vi "数据编码.vi"(0 "table输入":string(combo), 1 "仪器参数上传时间":enum16{"精确到小时", "原始时间"}(ring), 5 "错误常量 2":errorcluster caption="错误输入", 7 "仪器参数":string[](array[string]), 9 "QN":string, 11 "参数":string, 13 "MN":string, 14 "PW":string) -> (4 "错误常量":errorcluster caption="错误输出", 15 "通讯包字符串":string)   [LabVIEW 2016, in "数据传输系统-05.lvlib"]
panel:
  out "核查数据发送次数":i32
  out "小时数据发送次数":i32
  out "长度":i32
  in  "数据块":T1
  out "通讯包":T2={"包头（2）"="##", "数据段长度（4）"="", "数据段"="", "CRC校验"="", "包尾"=""}
  # "范例代码：\n\n##0101QN=20160801085857223;ST=32;CN=1062;PW=100000;MN=010000A8900016F000169DC0;Flag=5\n;CP=&&RtdInterval=30&&1C80\\r\\n"
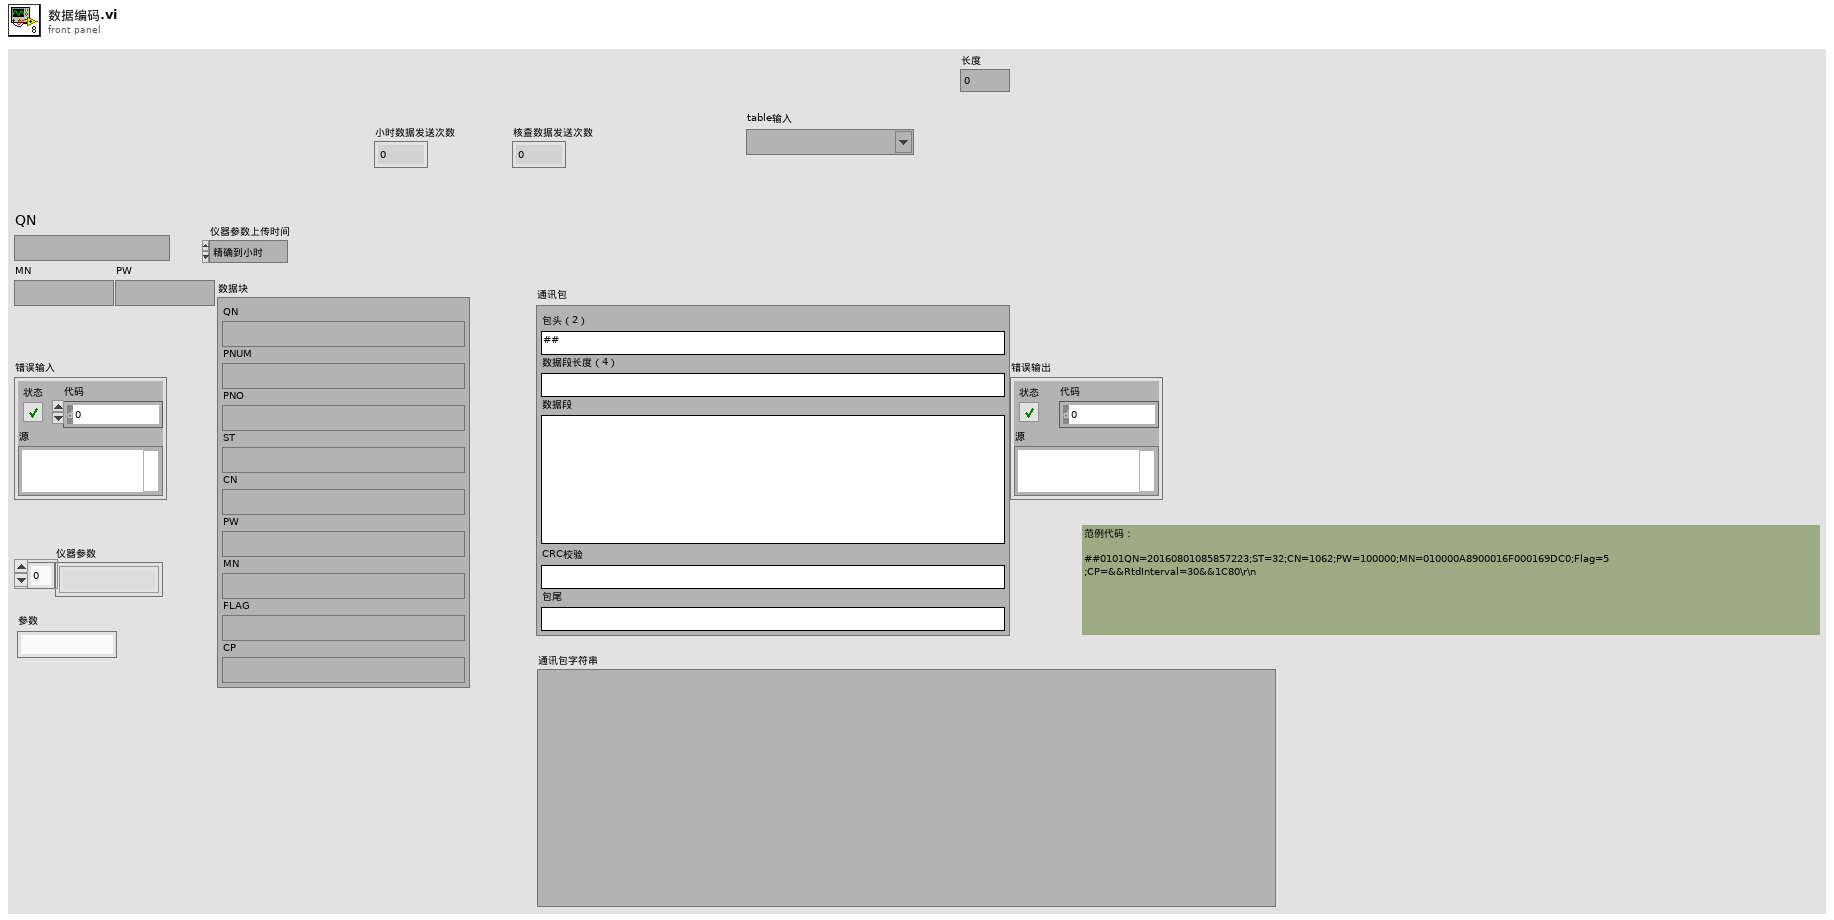
[diagram p1: front panel]
types:
  T1 = cluster{"QN":string, "ST":string, "CN":string, "PW":string, "MN":string, "FLAG":string, "PNUM":string, "PNO":string, "CP":string}
  T2 = cluster{"包头（2）":string, "数据段长度（4）":string, "数据段":string, "CRC校验":string, "包尾":string}
  T3 = cluster{"PH":string[][], "CODCr":string[][], "氨氮":string[][], "CODMn":string[][], "总氮":string[][], "总磷":string[][], "电导率":string[][], "水温":string[][], "DO":string[][], "浊度":string[][], "叶绿素":string[][], "藻密度":string[][], "铜":string[][], "盐度":string[][], "水位":string[][], "流速":string[][], "瞬时流量":string[][], "累积流量":string[][], "亚硝酸盐":string[][], "硫化物":string[][], "ORP":string[][], "铅":string[][], "镉":string[][], "锌":string[][], "镍":string[][], "锰":string[][], "汞":string[][], "气温":string[][], "气压":string[][], "风速":string[][], "风向":string[][], "盐度 2":string[][], "磷酸盐":string[][], "硝氮":string[][], "氟化物":string[][]}
  T4 = enum16{"小时数据", "实时数据", "平行样测试", "集成干预测试", "加标回收测试", "核查数据", "空白零点跨度数据", "提取小时数据", "提取实时数据"}
  T5 = enum16{"小时数据", "实时数据", "平行样测试", "集成干预测试", "加标回收测试", "核查数据", "空白零点跨度数据", "提取小时数据", "提取实时数据", "操作日志"}
  T6 = enum16{"小时数据", "实时数据", "平行样测试", "集成干预测试", "加标回收测试", "核查数据", "空白零点跨度数据", "提取小时数据", "提取实时数据", "操作日志", "仪器参数", "3090仪器参数", "提取仪器参数", "报警信息"}
  T7 = cluster{"CODMn":string, "CODCr":string, "DO":string, "铜":string, "PH":string, "氨氮":string, "比电导率":string, "水温":string, "COD":string, "浊度":string, "总氮":string, "总磷":string, "叶绿素a":string, "藻密度":string, "水位":string, "流速":string, "瞬时流量":string, "累积流量":string, "亚硝酸盐":string, "硫化物":string, "ORP":string, "铅":string, "镉":string, "锌":string, "镍":string, "锰":string, "汞":string, "气温":string, "气压":string, "风速":string, "风向":string, "盐度":string, "磷酸盐":string, "硝氮":string, "氟化物":string}
  T8 = cluster{"CODMn":dbl, "CODCr":dbl, "DO":dbl, "铜":dbl, "PH":dbl, "氨氮":dbl, "比电导率":dbl, "水温":dbl, "COD":dbl, "浊度":dbl, "总氮":dbl, "总磷":dbl, "叶绿素a":dbl, "藻密度":dbl, "水位":dbl, "流速":dbl, "瞬时流量":dbl, "累积流量":dbl, "亚硝酸盐":dbl, "硫化物":dbl, "ORP":dbl, "铅":dbl, "镉":dbl, "锌":dbl, "镍":dbl, "锰":dbl, "汞":dbl, "气温":dbl, "气压":dbl, "风速":dbl, "风向":dbl, "盐度":dbl, "磷酸盐":dbl, "硝氮":dbl, "氟化物":dbl}
  T9 = typedef "LVDateTimeRec.ctl" = cluster{"秒数的小数部分":dbl, "秒":i32, "分":i32, "时":i32, "日":i32, "月":i32, "年":i32, "天数（周）":i32, "天数（年）":i32, "DST":i32}
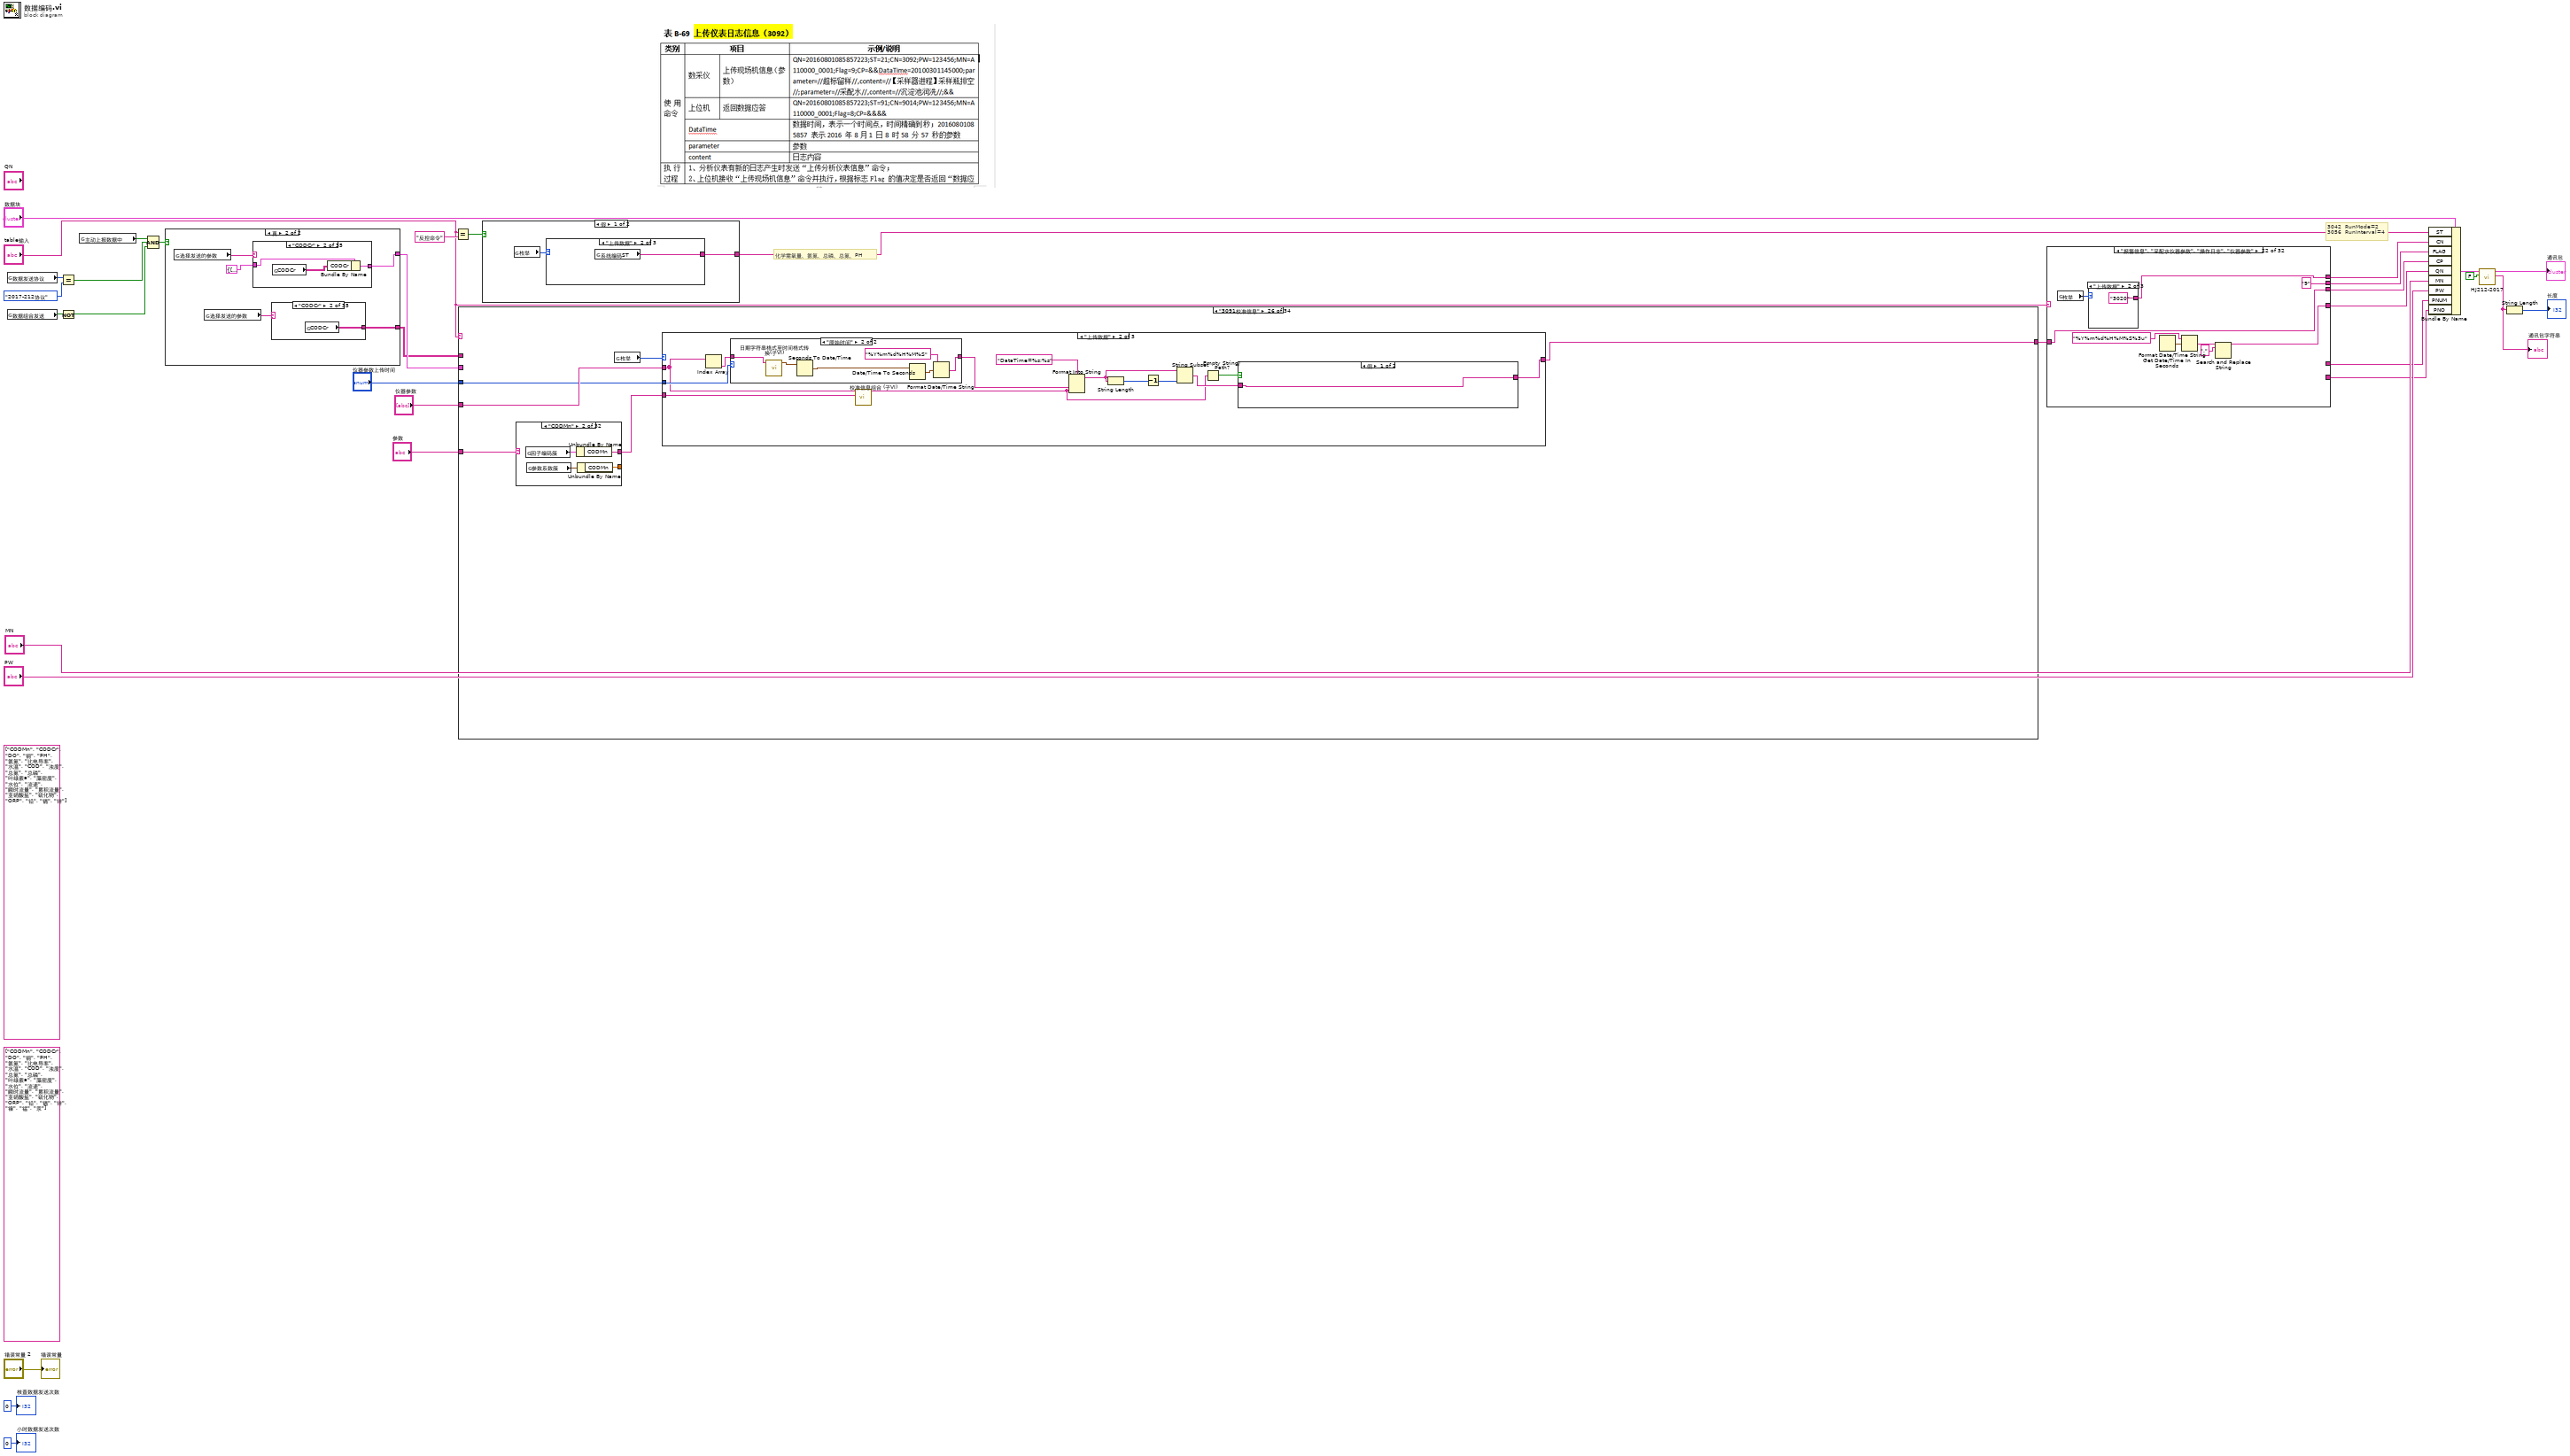
[diagram p0: block diagram]
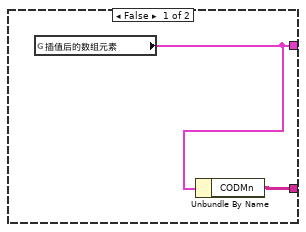
[diagram p2: hidden frame]
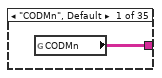
[diagram p3: hidden frame]
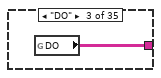
[diagram p4: hidden frame]
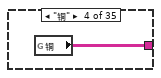
[diagram p5: hidden frame]
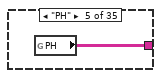
[diagram p6: hidden frame]
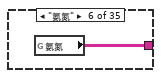
[diagram p7: hidden frame]
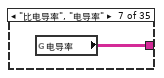
[diagram p8: hidden frame]
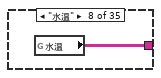
[diagram p9: hidden frame]
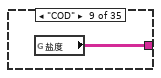
[diagram p10: hidden frame]
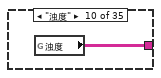
[diagram p11: hidden frame]
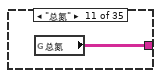
[diagram p12: hidden frame]
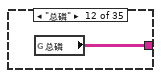
[diagram p13: hidden frame]
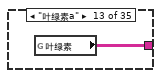
[diagram p14: hidden frame]
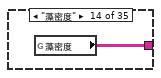
[diagram p15: hidden frame]
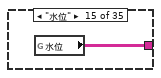
[diagram p16: hidden frame]
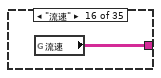
[diagram p17: hidden frame]
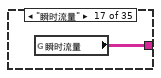
[diagram p18: hidden frame]
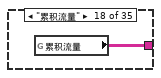
[diagram p19: hidden frame]
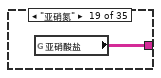
[diagram p20: hidden frame]
diagram:
  (unwired) string[] ["CODMn", "CODCr", "DO", "铜", "PH", "氨氮", "比电导率", "水温", "COD", "浊度", "总氮", "总磷", "叶绿素a", "藻密度", "水位", "流速", "瞬时流量", "累积流量", "亚硝酸盐", "硫化物", "ORP", "铅", "镉", "锌"] ("数组")
  (unwired) string[] ["CODMn", "CODCr", "DO", "铜", "PH", "氨氮", "比电导率", "水温", "COD", "浊度", "总氮", "总磷", "叶绿素a", "藻密度", "水位", "流速", "瞬时流量", "累积流量", "亚硝酸盐", "硫化物", "ORP", "铅", "镉", "锌", "镍", "锰", "汞"] ("数组")
  # "化学需氧量、氨氮、总磷、总氮、PH"
  # "3042  RunMode=2\n3056  RunInterval=4"
  n1 = global read "断电保存全局.vi" "数据发送协议"() -> (w11:enum16{"2005-212协议", "2017-212协议"})
  n2 = global read "断电保存全局.vi" "数据组合发送"() -> (w13:bool)
  n3 = Equal?(x=w11, y=enum16{"2005-212协议", "2017-212协议"}."2017-212协议" ("数据发送版本")) -> (x = y?=w14:bool)
  n4 = Not(x=w13) -> (.not. x?=w12:bool)
  n5 = global read "全局 数据发送重叠.vi" "主动上报数据中"() -> (w18:bool)
  n6 = Compound Arithmetic op=AND ("复合运算")(w18, w14, w12) -> (w15:bool)
  n7 = case shown="真" w15 {
    tunnel: [w36 w40] -> w9
    tunnel: [w35 w38] -> w7
    frame False {
      n8 = global read "插值后的新数组.vi" "插值后的数组元素"() -> (w36:T3)
      n9 = Unbundle By Name(w36) -> ("CODMn"=w35:string[][])
    }
    frame True {
      n10 = global read "全局 水样时间.vi" "选择发送的参数"() -> (w41:string)
      n11 = global read "全局 水样时间.vi" "选择发送的参数"() -> (w39:string)
      n12 = case shown="\"CODCr\"" w41 {
        tunnel: T3 {"PH"=[], "CODCr"=[], "氨氮"=[], "CODMn"=[], "总氮"=[], "总磷"=[], "电导率"=[], "水温"=[], "DO"=[], "浊度"=[], "叶绿素"=[], "藻密度"=[], "铜"=[], "盐度"=[], "水位"=[], "流速"=[], "瞬时流量"=[], "累积流量"=[], "亚硝酸盐"=[], "硫化物"=[], "ORP"=[], "铅"=[], "镉"=[], "锌"=[], "镍"=[], "锰"=[], "汞"=[], "气温"=[], "气压"=[], "风速"=[], "风向"=[], "盐度 2"=[], "磷酸盐"=[], "硝氮"=[], "氟化物"=[]} ("插值后的数组元素") -> [w78 w82 w85 w88 w91 w94 w97 w100 w103 w106 w109 w112 w115 w117 w121 w124 w126 w129 w132 w135 w138 w141 w144 w147 w150 w153 w156 w159 w162 w165 w168 w171 w174 w177 w180]
        tunnel: [w77 w80 w83 w86 w89 w92 w96 w99 w101 w104 w107 w110 w113 w116 w119 w122 w125 w128 w131 w134 w137 w140 w143 w146 w149 w152 w155 w158 w161 w164 w167 w170 w173 w176 w179] -> w40
        frame "CODMn", Default {
          n13 = global read "全局 所有参数.vi" "CODMn"() -> (w79:string[][])
          n14 = Bundle By Name(cluster=w78, "CODMn"=w79) -> (w77:T3)
        }
        frame "CODCr" {
          n15 = global read "全局 所有参数.vi" "CODCr"() -> (w81:string[][])
          n16 = Bundle By Name(cluster=w82, "CODCr"=w81) -> (w80:T3)
        }
        frame "DO" {
          n17 = global read "全局 所有参数.vi" "DO"() -> (w84:string[][])
          n18 = Bundle By Name(cluster=w85, "DO"=w84) -> (w83:T3)
        }
        frame "铜" {
          n19 = global read "全局 所有参数.vi" "铜"() -> (w87:string[][])
          n20 = Bundle By Name(cluster=w88, "铜"=w87) -> (w86:T3)
        }
        frame "PH" {
          n21 = global read "全局 所有参数.vi" "PH"() -> (w90:string[][])
          n22 = Bundle By Name(cluster=w91, "PH"=w90) -> (w89:T3)
        }
        frame "氨氮" {
          n23 = global read "全局 所有参数.vi" "氨氮"() -> (w93:string[][])
          n24 = Bundle By Name(cluster=w94, "氨氮"=w93) -> (w92:T3)
        }
        frame "比电导率", "电导率" {
          n25 = global read "全局 所有参数.vi" "电导率"() -> (w95:string[][])
          n26 = Bundle By Name(cluster=w97, "电导率"=w95) -> (w96:T3)
        }
        frame "水温" {
          n27 = global read "全局 所有参数.vi" "水温"() -> (w98:string[][])
          n28 = Bundle By Name(cluster=w100, "水温"=w98) -> (w99:T3)
        }
        frame "COD" {
          n29 = global read "全局 所有参数.vi" "盐度"() -> (w102:string[][])
          n30 = Bundle By Name(cluster=w103, "盐度"=w102) -> (w101:T3)
        }
        frame "浊度" {
          n31 = global read "全局 所有参数.vi" "浊度"() -> (w105:string[][])
          n32 = Bundle By Name(cluster=w106, "浊度"=w105) -> (w104:T3)
        }
        frame "总氮" {
          n33 = global read "全局 所有参数.vi" "总氮"() -> (w108:string[][])
          n34 = Bundle By Name(cluster=w109, "总氮"=w108) -> (w107:T3)
        }
        frame "总磷" {
          n35 = global read "全局 所有参数.vi" "总磷"() -> (w111:string[][])
          n36 = Bundle By Name(cluster=w112, "总磷"=w111) -> (w110:T3)
        }
        frame "叶绿素a" {
          n37 = global read "全局 所有参数.vi" "叶绿素"() -> (w114:string[][])
          n38 = Bundle By Name(cluster=w115, "叶绿素"=w114) -> (w113:T3)
        }
        frame "藻密度" {
          n39 = global read "全局 所有参数.vi" "藻密度"() -> (w118:string[][])
          n40 = Bundle By Name(cluster=w117, "藻密度"=w118) -> (w116:T3)
        }
        frame "水位" {
          n41 = global read "全局 所有参数.vi" "水位"() -> (w120:string[][])
          n42 = Bundle By Name(cluster=w121, "水位"=w120) -> (w119:T3)
        }
        frame "流速" {
          n43 = global read "全局 所有参数.vi" "流速"() -> (w123:string[][])
          n44 = Bundle By Name(cluster=w124, "流速"=w123) -> (w122:T3)
        }
        frame "瞬时流量" {
          n45 = global read "全局 所有参数.vi" "瞬时流量"() -> (w127:string[][])
          n46 = Bundle By Name(cluster=w126, "瞬时流量"=w127) -> (w125:T3)
        }
        frame "累积流量" {
          n47 = global read "全局 所有参数.vi" "累积流量"() -> (w130:string[][])
          n48 = Bundle By Name(cluster=w129, "累积流量"=w130) -> (w128:T3)
        }
        frame "亚硝氮" {
          n49 = global read "全局 所有参数.vi" "亚硝酸盐"() -> (w133:string[][])
          n50 = Bundle By Name(cluster=w132, "亚硝酸盐"=w133) -> (w131:T3)
        }
        frame "硫化物" {
          n51 = global read "全局 所有参数.vi" "硫化物"() -> (w136:string[][])
          n52 = Bundle By Name(cluster=w135, "硫化物"=w136) -> (w134:T3)
        }
        frame "ORP" {
          n53 = global read "全局 所有参数.vi" "ORP"() -> (w139:string[][])
          n54 = Bundle By Name(cluster=w138, "ORP"=w139) -> (w137:T3)
        }
        frame "铅" {
          n55 = global read "全局 所有参数.vi" "铅"() -> (w142:string[][])
          n56 = Bundle By Name(cluster=w141, "铅"=w142) -> (w140:T3)
        }
        frame "镉" {
          n57 = global read "全局 所有参数.vi" "镉"() -> (w145:string[][])
          n58 = Bundle By Name(cluster=w144, "镉"=w145) -> (w143:T3)
        }
        frame "锌" {
          n59 = global read "全局 所有参数.vi" "锌"() -> (w148:string[][])
          n60 = Bundle By Name(cluster=w147, "锌"=w148) -> (w146:T3)
        }
        frame "镍" {
          n61 = global read "全局 所有参数.vi" "镍"() -> (w151:string[][])
          n62 = Bundle By Name(cluster=w150, "镍"=w151) -> (w149:T3)
        }
        frame "锰" {
          n63 = global read "全局 所有参数.vi" "锰"() -> (w154:string[][])
          n64 = Bundle By Name(cluster=w153, "锰"=w154) -> (w152:T3)
        }
        frame "汞" {
          n65 = global read "全局 所有参数.vi" "汞"() -> (w157:string[][])
          n66 = Bundle By Name(cluster=w156, "汞"=w157) -> (w155:T3)
        }
        frame "气温" {
          n67 = global read "全局 所有参数.vi" "气温"() -> (w160:string[][])
          n68 = Bundle By Name(cluster=w159, "气温"=w160) -> (w158:T3)
        }
        frame "气压" {
          n69 = global read "全局 所有参数.vi" "气压"() -> (w163:string[][])
          n70 = Bundle By Name(cluster=w162, "气压"=w163) -> (w161:T3)
        }
        frame "风速" {
          n71 = global read "全局 所有参数.vi" "风速"() -> (w166:string[][])
          n72 = Bundle By Name(cluster=w165, "风速"=w166) -> (w164:T3)
        }
        frame "风向" {
          n73 = global read "全局 所有参数.vi" "风向"() -> (w169:string[][])
          n74 = Bundle By Name(cluster=w168, "风向"=w169) -> (w167:T3)
        }
        frame "盐度" {
          n75 = global read "全局 所有参数.vi" "盐度 2"() -> (w172:string[][])
          n76 = Bundle By Name(cluster=w171, "盐度 2"=w172) -> (w170:T3)
        }
        frame "磷酸盐" {
          n77 = global read "全局 所有参数.vi" "磷酸盐"() -> (w175:string[][])
          n78 = Bundle By Name(cluster=w174, "磷酸盐"=w175) -> (w173:T3)
        }
        frame "硝氮" {
          n79 = global read "全局 所有参数.vi" "硝氮"() -> (w178:string[][])
          n80 = Bundle By Name(cluster=w177, "硝氮"=w178) -> (w176:T3)
        }
        frame "氟化物" {
          n81 = global read "全局 所有参数.vi" "氟化物"() -> (w181:string[][])
          n82 = Bundle By Name(cluster=w180, "氟化物"=w181) -> (w179:T3)
        }
      }
      n83 = case shown="\"CODCr\"" w39 {
        tunnel: [w42 w43 w44 w45 w46 w47 w48 w49 w50 w51 w52 w53 w54 w55 w56 w57 w58 w59 w60 w61 w62 w63 w64 w65 w66 w67 w68 w69 w70 w71 w72 w73 w74 w75 w76] -> w38
        frame "CODMn", Default {
          n84 = global read "全局 所有参数.vi" "CODMn"() -> (w42:string[][])
        }
        frame "CODCr" {
          n85 = global read "全局 所有参数.vi" "CODCr"() -> (w43:string[][])
        }
        frame "DO" {
          n86 = global read "全局 所有参数.vi" "DO"() -> (w44:string[][])
        }
        frame "铜" {
          n87 = global read "全局 所有参数.vi" "铜"() -> (w45:string[][])
        }
        frame "PH" {
          n88 = global read "全局 所有参数.vi" "PH"() -> (w46:string[][])
        }
        frame "氨氮" {
          n89 = global read "全局 所有参数.vi" "氨氮"() -> (w47:string[][])
        }
        frame "比电导率", "电导率" {
          n90 = global read "全局 所有参数.vi" "电导率"() -> (w48:string[][])
        }
        frame "水温" {
          n91 = global read "全局 所有参数.vi" "水温"() -> (w49:string[][])
        }
        frame "COD" {
          n92 = global read "全局 所有参数.vi" "盐度"() -> (w50:string[][])
        }
        frame "浊度" {
          n93 = global read "全局 所有参数.vi" "浊度"() -> (w51:string[][])
        }
        frame "总氮" {
          n94 = global read "全局 所有参数.vi" "总氮"() -> (w52:string[][])
        }
        frame "总磷" {
          n95 = global read "全局 所有参数.vi" "总磷"() -> (w53:string[][])
        }
        frame "叶绿素a" {
          n96 = global read "全局 所有参数.vi" "叶绿素"() -> (w54:string[][])
        }
        frame "藻密度" {
          n97 = global read "全局 所有参数.vi" "藻密度"() -> (w55:string[][])
        }
        frame "水位" {
          n98 = global read "全局 所有参数.vi" "水位"() -> (w56:string[][])
        }
        frame "流速" {
          n99 = global read "全局 所有参数.vi" "流速"() -> (w57:string[][])
        }
        frame "瞬时流量" {
          n100 = global read "全局 所有参数.vi" "瞬时流量"() -> (w58:string[][])
        }
        frame "累积流量" {
          n101 = global read "全局 所有参数.vi" "累积流量"() -> (w59:string[][])
        }
        frame "亚硝氮" {
          n102 = global read "全局 所有参数.vi" "亚硝酸盐"() -> (w60:string[][])
        }
        frame "硫化物" {
          n103 = global read "全局 所有参数.vi" "硫化物"() -> (w61:string[][])
        }
        frame "ORP" {
          n104 = global read "全局 所有参数.vi" "ORP"() -> (w62:string[][])
        }
        frame "铅" {
          n105 = global read "全局 所有参数.vi" "铅"() -> (w63:string[][])
        }
        frame "镉" {
          n106 = global read "全局 所有参数.vi" "镉"() -> (w64:string[][])
        }
        frame "锌" {
          n107 = global read "全局 所有参数.vi" "锌"() -> (w65:string[][])
        }
        frame "镍" {
          n108 = global read "全局 所有参数.vi" "镍"() -> (w66:string[][])
        }
        frame "锰" {
          n109 = global read "全局 所有参数.vi" "锰"() -> (w67:string[][])
        }
        frame "汞" {
          n110 = global read "全局 所有参数.vi" "汞"() -> (w68:string[][])
        }
        frame "气温" {
          n111 = global read "全局 所有参数.vi" "气温"() -> (w69:string[][])
        }
        frame "气压" {
          n112 = global read "全局 所有参数.vi" "气压"() -> (w70:string[][])
        }
        frame "风速" {
          n113 = global read "全局 所有参数.vi" "风速"() -> (w71:string[][])
        }
        frame "风向" {
          n114 = global read "全局 所有参数.vi" "风向"() -> (w72:string[][])
        }
        frame "盐度" {
          n115 = global read "全局 所有参数.vi" "盐度 2"() -> (w73:string[][])
        }
        frame "磷酸盐" {
          n116 = global read "全局 所有参数.vi" "磷酸盐"() -> (w74:string[][])
        }
        frame "硝氮" {
          n117 = global read "全局 所有参数.vi" "硝氮"() -> (w75:string[][])
        }
        frame "氟化物" {
          n118 = global read "全局 所有参数.vi" "氟化物"() -> (w76:string[][])
        }
      }
    }
  }
  n119 = Equal?(x="table输入", y="反控命令") -> (x = y?=w24:bool)
  n120 = case shown="\"3091校准信息\"" "table输入" {
    tunnel: [w183 w190 w204 w247 w270 _ w284 w293 w304 w454 w485 w536 w583 w634 w663 w695 w726 w752 w781 w810 w847 w880 w913 w949 w1110 w1152 w1313 w1341 w1364 w1397 w1420 w1431 w1439 w1449] -> w19
    tunnel: w7 -> [_ _ _ _ _ _ _ _ w301 w453 _ _ _ w633 w664 w690 w721 w753 w780 w809 w846 _ _ _ _ _ w1312 _ w1363 _ _ _ _ _]
    tunnel: w9 -> [_ _ _ _ _ _ _ _ w302 w455 _ _ _ w629 w659 w691 w722 w751 w779 w808 w842 _ _ _ _ _ w1308 w1339 w1359 _ _ _ _ _]
    tunnel: "仪器参数" -> [_ _ _ _ _ _ _ _ _ _ _ _ _ _ _ _ _ _ _ _ _ _ _ w945 w1108 w1148 _ _ _ _ _ _ _ _]
    tunnel: "参数" -> [_ _ _ _ _ _ _ _ _ _ _ _ _ _ _ _ _ _ _ _ _ _ _ w947 _ w1150 _ _ _ _ _ _ _ _]
    tunnel: "仪器参数上传时间" -> [_ _ _ _ _ _ _ _ _ _ _ _ _ _ _ _ _ _ _ _ _ _ _ w944 w1107 w1147 _ _ _ _ _ _ _ _]
    frame "反控命令" {
      n121 = global read "全局 反控命令枚举.vi" "反控命令枚举"() -> (w182:enum16{"返回请求应答", "返回执行结果"})
      n122 = case shown="\"返回执行结果\"" w182 {
        tunnel: ["QnRtn=1" w186] -> w183
        frame "返回请求应答", Default {
        }
        frame "返回执行结果" {
          n123 = global read "全局 反控命令枚举.vi" "执行结果定义"() -> (w187:u16)
          n124 = Number To Decimal String(number=w187) -> (decimal integer string=w185:string)  [unwired: 1 in]
          n125 = Concatenate Strings("ExeRtn=", w185) -> (w186:string)
        }
      }
    }
    frame "超标留样返回" {
      n126 = global read "全局1.vi" "枚举"() -> (w189:enum16{"返回请求应答", "上传数据", "返回执行结果"})
      n127 = case shown="\"返回请求应答\", 默认" w189 {
        tunnel: ["QnRtn=1" w192 "ExeRtn=1"] -> w190
        frame "返回请求应答", Default {
        }
        frame "上传数据" {
          n128 = global read "全局1.vi" "register values"() -> (w201:u16[])
          n129 = Get Date/Time In Seconds() -> (seconds since 1Jan1904=w199:timestamp)
          n130 = Index Array(array=w201, index=7 ("索引")) -> (element=w194:u16)
          n131 = Format Date/Time String(time format string (%c)="%Y%m%d%H%M%S" ("时间格式字符串(%c)"), seconds (now)=w199) -> (date/time string=w197:string)  [unwired: 1 in]
          n132 = Number To Decimal String(number=w194) -> (decimal integer string=w195:string)  [unwired: 1 in]
          n133 = Format Into String(format string="VaseNo=%s" ("格式字符串"), w195) -> (resulting string=w193:string)  [unwired: 2 in, 1 out]
          n134 = Format Into String(format string="DataTime=%s;%s" ("格式字符串"), w197, w193) -> (resulting string=w192:string)  [unwired: 2 in, 1 out]
        }
        frame "返回执行结果" {
        }
      }
    }
    frame "提取经纬度环境信息" {
      # "BDS纬度"
      # "BDS纬度"
      # "GPS纬度"
      # "GPS经度"
      # "湿度"
      # "温度"
      # "电压"
      # "时间"
      n135 = global read "全局1.vi" "枚举"() -> (w205:enum16{"返回请求应答", "上传数据", "返回执行结果"})
      n136 = case shown="\"上传数据\"" w205 {
        tunnel: ["QnRtn=1" w218 "ExeRtn=1"] -> w204
        frame "返回请求应答", Default {
        }
        frame "上传数据" {
          n137 = global read "全局 环境参数.vi" "环境参数"() -> (w208:string[][])
          n138 = global read "全局 环境参数.vi" "columns输出"() -> (w215:string[])
          n139 = Index Array(array=w208, index (row)=0 ("索引 (行)")) -> (element=w211:string[])  [unwired: 1 in]
          n140 = Get Date/Time In Seconds() -> (seconds since 1Jan1904=w220:timestamp)
          n141 = Array Subset(array=w215, index=1 ("索引")) -> (w216:string[])  [unwired: 1 in]
          n142 = for {
            tunnel: w216 -> [w224] mode=indexing
            tunnel: [w223] -> w217 mode=indexing
            n143 = case shown="\"BDS经度\"" w224 {
              tunnel: ["" "Volt=%s;" "Temp=%s;" ("格式字符串") "Hum=%s;" ("格式字符串") "Lng=%s;" "Lat=%s;" "Lng2=%s;" "Lat2=%s;"] -> w223
              frame "假", Default {
              }
              frame "电压" {
              }
              frame "室温" {
              }
              frame "湿度" {
              }
              frame "GPS经度" {
              }
              frame "GPS纬度" {
              }
              frame "BDS经度" {
              }
              frame "BDS纬度" {
              }
            }
          }
          n144 = Format Date/Time String(time format string (%c)="%Y%m%d%H%M%S" ("时间格式字符串(%c)"), seconds (now)=w220) -> (date/time string=w219:string)  [unwired: 1 in]
          n145 = Array Subset(array=w211, index=1 ("索引")) -> (w213:string[])  [unwired: 1 in]
          n146 = for {
            shift-right: [w238] -> w207
            shift-left: "" -> [w237]
            tunnel: w217 -> [w236] mode=indexing
            tunnel: w213 -> [w234] mode=indexing
            n147 = Empty String/Path?(string/path=w234) -> (empty?=w240:bool)
            n148 = Fract/Exp String To Number(string=w234) -> (number=w235:dbl)  [unwired: 3 in, 1 out]
            n149 = Number To Fractional String(number=w235) -> (F-format string=w233:string)  [unwired: 3 in]
            n150 = case shown="假" w240 {
              tunnel: [w243 w244] -> w239
              tunnel: w236 -> [w242 _]
              tunnel: w233 -> [w241 _]
              tunnel: w233 -> [_ w244]
              frame False {
                n151 = Format Into String(format string=w242, w241) -> (resulting string=w243:string)  [unwired: 2 in, 1 out]
              }
              frame True {
              }
            }
            n152 = Concatenate Strings(w237, w239) -> (w238:string)
          }
          n153 = Format Into String(format string="DataTime=%s;%s" ("格式字符串"), w219, w207) -> (resulting string=w218:string)  [unwired: 2 in, 1 out]
        }
        frame "返回执行结果" {
        }
      }
    }
    frame "提取现场系统信息" {
      n154 = global read "全局1.vi" "枚举"() -> (w246:enum16{"返回请求应答", "上传数据", "返回执行结果"})
      n155 = case shown="\"上传数据\"" w246 {
        tunnel: ["QnRtn=1" w267 "ExeRtn=1"] -> w247
        frame "返回请求应答", Default {
        }
        frame "上传数据" {
          n156 = global read "全局1.vi" "register values"() -> (w266:u16[])
          n157 = Index Array(array=w266, index #1=0 ("索引"), index #2=6 ("索引")) -> (element #1=w262:u16, element #2=w249:u16)
          n158 = Number To Decimal String(number=w262) -> (decimal integer string=w264:string)  [unwired: 1 in]
          n159 = Number To Decimal String(number=w249) -> (decimal integer string=w258:string)  [unwired: 1 in]
          n160 = Get Date/Time In Seconds() -> (seconds since 1Jan1904=w252:timestamp)
          n161 = Format Date/Time String(time format string (%c)="%Y%m%d%H%M%S%u" ("时间格式字符串(%c)"), seconds (now)=w252) -> (date/time string=w255:string)  [unwired: 1 in]
          n162 = Format Into String(format string="RunMode=%s;" ("格式字符串"), w264) -> (resulting string=w261:string)  [unwired: 2 in, 1 out]
          n163 = Format Into String(format string="RunInterval=%s;" ("格式字符串"), w258) -> (resulting string=w259:string)  [unwired: 2 in, 1 out]
          n164 = Search and Replace String(input string=w255, search string="." ("搜索字符串")) -> (result string=w251:string)  [unwired: 6 in, 3 out]
          n165 = Format Into String(format string="SystemTime=%s;" ("格式字符串"), w251) -> (resulting string=w256:string)  [unwired: 2 in, 1 out]
          n166 = Concatenate Strings(w261, w259, w256) -> (w267:string)
        }
        frame "返回执行结果" {
        }
      }
    }
    frame "提取监测仪表时间" {
      n167 = global read "全局1.vi" "枚举"() -> (w269:enum16{"返回请求应答", "上传数据", "返回执行结果"})
      n168 = case shown="\"上传数据\"" w269 {
        tunnel: ["QnRtn=1" w282 "ExeRtn=1"] -> w270
        frame "返回请求应答", Default {
        }
        frame "上传数据" {
          n169 = global read "全局 提取仪器参数.vi" "仪器编码"() -> (w272:string)
          n170 = Format Into String(format string="PolId=%s;" ("格式字符串"), w272) -> (resulting string=w280:string)  [unwired: 2 in, 1 out]
          n171 = Get Date/Time In Seconds() -> (seconds since 1Jan1904=w275:timestamp)
          n172 = Format Date/Time String(time format string (%c)="%Y%m%d%H%M%S%u" ("时间格式字符串(%c)"), seconds (now)=w275) -> (date/time string=w278:string)  [unwired: 1 in]
          n173 = Search and Replace String(input string=w278, search string="." ("搜索字符串")) -> (result string=w274:string)  [unwired: 6 in, 3 out]
          n174 = Format Into String(format string="SystemTime=%s;" ("格式字符串"), w274) -> (resulting string=w273:string)  [unwired: 2 in, 1 out]
          n175 = Concatenate Strings(w280, w273) -> (w282:string)
        }
        frame "返回执行结果" {
        }
      }
    }
    frame "心跳包", Default {
    }
    frame "提取数采仪时间" {
      (unwired) ""
      n176 = global read "全局1.vi" "枚举"() -> (w285:enum16{"返回请求应答", "上传数据", "返回执行结果"})
      n177 = case shown="\"上传数据\"" w285 {
        tunnel: ["QnRtn=1" w287 "ExeRtn=1"] -> w284
        frame "返回请求应答", Default {
        }
        frame "上传数据" {
          n178 = Get Date/Time In Seconds() -> (seconds since 1Jan1904=w291:timestamp)
          n179 = Format Date/Time String(time format string (%c)="%Y%m%d%H%M%S" ("时间格式字符串(%c)"), seconds (now)=w291) -> (date/time string=w288:string)  [unwired: 1 in]
          n180 = Concatenate Strings("SystemTime=", w288) -> (w287:string)
        }
        frame "返回执行结果" {
        }
      }
    }
    frame "提取实时数据间隔" {
      (unwired) ""
      n181 = global read "全局1.vi" "枚举"() -> (w294:enum16{"返回请求应答", "上传数据", "返回执行结果"})
      n182 = case shown="\"上传数据\"" w294 {
        tunnel: ["QnRtn=1" w298 "ExeRtn=1"] -> w293
        frame "返回请求应答", Default {
        }
        frame "上传数据" {
          n183 = global read "实时数据发送间隔全局.vi" "实时数据发送间隔"() -> (w297:u32)
          n184 = Number To Decimal String(number=w297) -> (decimal integer string=w296:string)  [unwired: 1 in]
          n185 = Concatenate Strings("RtdInterval=", w296) -> (w298:string)
        }
        frame "返回执行结果" {
        }
      }
    }
    frame "实时数据" {
      # "包含质控数据主动上传"
      n186 = global read "全局 实时数据参数.vi" "实时数据参数"() -> (w303:string)
      n187 = case shown="\"核查数据\"" w303 {
        tunnel: [w307 w332 w357 w388 w412 w433] -> w304
        tunnel: w302 -> [w306 w331 w356 w386 w410 w431]
        tunnel: w301 -> [w305 w330 w355 w385 w409 w430]
        frame "水样测试", Default {
          n188 = global read "全局1.vi" "枚举"() -> (w308:enum16{"返回请求应答", "上传数据", "返回执行结果"})
          n189 = case shown="\"上传数据\"" w308 {
            tunnel: ["QnRtn=1" w326 "ExeRtn=1"] -> w307
            tunnel: w306 -> [_ w312 _]
            tunnel: w305 -> [_ w310 _]
            frame "返回请求应答", Default {
            }
            frame "上传数据" {
              n190 = call "数据发送组合-20200825 (子VI).vi"("枚举"=T4."实时数据", "插值后的数组元素"=w312) -> ("字符串"=w313:string)  [unwired: 9 in]
              n191 = global read "全局 小时数据发送次数.vi" "小时数据发送次数"() -> (w324:i32)
              n192 = Empty String/Path?(string/path=w313) -> (empty?=w325:bool)
              n193 = Index Array(array=w310, index (row)=w324) -> (element=w323:string[])  [unwired: 1 in]
              n194 = Index Array(array=w323, index=0 ("索引")) -> (element=w321:string)
              n195 = call "规范时间戳.vi"("字符串"=w321) -> ("result string"=w319:string)  [unwired: 10 in]
              n196 = Format Into String(format string="DataTime=%s;", w319) -> (resulting string=w318:string)  [unwired: 2 in, 1 out]
              n197 = Concatenate Strings(w318, w313) -> (w315:string)
              n198 = String Length(string=w315) -> (length=w317:i32)
              n199 = Decrement(x=w317) -> (x-1=w316:i32)
              n200 = String Subset(string=w315, length (rest)=w316) -> (substring=w314:string)  [unwired: 1 in]
              n201 = case shown="假" w325 {
                tunnel: [w327 ""] -> w326
                tunnel: w314 -> [w327 _]
                frame False {
                }
                frame True {
                }
              }
            }
            frame "返回执行结果" {
            }
          }
        }
        frame "平行样测试" {
          n202 = global read "全局1.vi" "枚举"() -> (w333:enum16{"返回请求应答", "上传数据", "返回执行结果"})
          n203 = case shown="\"上传数据\"" w333 {
            tunnel: ["QnRtn=1" w345 "ExeRtn=1"] -> w332
            tunnel: w330 -> [_ w339 _]
            tunnel: w331 -> [_ w336 _]
            frame "返回请求应答", Default {
            }
            frame "上传数据" {
              # "CODMn"
              n204 = call "数据发送组合-20200825 (子VI).vi"("枚举"=T4."平行样测试", "插值后的数组元素"=w336) -> ("字符串"=w335:string)  [unwired: 9 in]
              n205 = global read "全局 小时数据发送次数.vi" "小时数据发送次数"() -> (w338:i32)
              n206 = Index Array(array=w339, index (row)=w338) -> (element=w343:string[])  [unwired: 1 in]
              n207 = Index Array(array=w343, index=0 ("索引")) -> (element=w340:string)
              n208 = call "规范时间戳.vi"("字符串"=w340) -> ("result string"=w341:string)  [unwired: 10 in]
              n209 = Empty String/Path?(string/path=w340) -> (empty?=w344:bool)
              n210 = Format Into String(format string="DataTime=%s;%s" ("格式字符串"), w341, w335) -> (resulting string=w346:string)  [unwired: 2 in, 1 out]
              n211 = case shown="真" w344 {
                tunnel: [w350 ""] -> w345
                tunnel: w346 -> [w350 _]
                frame False {
                  n212 = global read "全局 小时数据发送次数.vi" "小时数据发送次数"() -> (w349:i32)
                  n213 = Increment(x=w349) -> (x+1=w348:i32)
                  n214 = global write "全局 小时数据发送次数.vi" "小时数据发送次数"(w348) -> ()
                }
                frame True {
                  n215 = global read "全局 小时数据发送次数.vi" "小时数据发送次数"() -> (w352:i32)
                  n216 = Increment(x=w352) -> (x+1=w351:i32)
                  n217 = global write "全局 小时数据发送次数.vi" "小时数据发送次数"(w351) -> ()
                }
              }
            }
            frame "返回执行结果" {
            }
          }
        }
        frame "集成干预测试" {
          n218 = global read "全局1.vi" "枚举"() -> (w358:enum16{"返回请求应答", "上传数据", "返回执行结果"})
          n219 = case shown="\"上传数据\"" w358 {
            tunnel: ["QnRtn=1" w371 "ExeRtn=1"] -> w357
            tunnel: w355 -> [_ w365 _]
            tunnel: w356 -> [_ w362 _]
            frame "返回请求应答", Default {
            }
            frame "上传数据" {
              # "CODMn"
              n220 = global read "全局 小时数据发送次数.vi" "小时数据发送次数"() -> (w364:i32)
              n221 = call "数据发送组合-20200825 (子VI).vi"("枚举"=T4."集成干预测试", "插值后的数组元素"=w362) -> ("字符串"=w361:string)  [unwired: 9 in]
              n222 = Index Array(array=w365, index (row)=w364) -> (element=w369:string[])  [unwired: 1 in]
              n223 = Index Array(array=w369, index=0 ("索引")) -> (element=w366:string)
              n224 = global read "断电保存全局.vi" "应用环境"() -> (w360:enum16{"STD", "GB212"})
              n225 = case shown="\"STD\", 默认" w360 {
                tunnel: [w375 w376] -> w367
                tunnel: w366 -> [w374 w377]
                frame "STD", Default {
                  n226 = call "规范时间戳.vi"("字符串"=w374) -> ("result string"=w375:string)  [unwired: 10 in]
                }
                frame "GB212" {
                  n227 = call "规范分钟数据时间戳.vi"("字符串"=w377) -> ("result string"=w376:string)  [unwired: 10 in]
                }
              }
              n228 = Empty String/Path?(string/path=w366) -> (empty?=w370:bool)
              n229 = Format Into String(format string="DataTime=%s;%s" ("格式字符串"), w367, w361) -> (resulting string=w372:string)  [unwired: 2 in, 1 out]
              n230 = case shown="假" w370 {
                tunnel: [w380 ""] -> w371
                tunnel: w372 -> [w380 _]
                frame False {
                  n231 = global read "全局 小时数据发送次数.vi" "小时数据发送次数"() -> (w379:i32)
                  n232 = Increment(x=w379) -> (x+1=w378:i32)
                  n233 = global write "全局 小时数据发送次数.vi" "小时数据发送次数"(w378) -> ()
                }
                frame True {
                  n234 = global read "全局 小时数据发送次数.vi" "小时数据发送次数"() -> (w382:i32)
                  n235 = Increment(x=w382) -> (x+1=w381:i32)
                  n236 = global write "全局 小时数据发送次数.vi" "小时数据发送次数"(w381) -> ()
                }
              }
            }
            frame "返回执行结果" {
            }
          }
        }
        frame "加标回收测试" {
          n237 = global read "全局1.vi" "枚举"() -> (w387:enum16{"返回请求应答", "上传数据", "返回执行结果"})
          n238 = case shown="\"上传数据\"" w387 {
            tunnel: ["QnRtn=1" w398 "ExeRtn=1"] -> w388
            tunnel: w385 -> [_ w393 _]
            tunnel: w386 -> [_ w395 _]
            frame "返回请求应答", Default {
            }
            frame "上传数据" {
              # "w01001-Check=63.0,w01001-WaterTime=20160801080000,w01001-Water=45.23,w01001-Chroma=1000,w01001-Volume=0.2,w01001-DVolume=200,w01003-Flag=N;"
              # "CODMn"
              n239 = global read "全局 小时数据发送次数.vi" "小时数据发送次数"() -> (w392:i32)
              n240 = call "加标回收数据组合 (子VI).vi"("小时数据发送次数"=w392, "数据"=w393, "污染物编码"="CODMn") -> ("datatime"=w391:string)  [unwired: 7 in, 1 out]
              n241 = call "规范时间戳.vi"("字符串"=w391) -> ("result string"=w400:string)  [unwired: 10 in]
              n242 = Empty String/Path?(string/path=w400) -> (empty?=w397:bool)
              n243 = call "数据发送组合-20200825 (子VI).vi"("枚举"=T4."加标回收测试", "插值后的数组元素"=w395) -> ("字符串"=w394:string)  [unwired: 9 in]
              n244 = Format Into String(format string="DataTime=%s;%s" ("格式字符串"), w400, w394) -> (resulting string=w399:string)  [unwired: 2 in, 1 out]
              n245 = case shown="真" w397 {
                tunnel: [w404 ""] -> w398
                tunnel: w399 -> [w404 _]
                frame False {
                  n246 = global read "全局 小时数据发送次数.vi" "小时数据发送次数"() -> (w403:i32)
                  n247 = Increment(x=w403) -> (x+1=w402:i32)
                  n248 = global write "全局 小时数据发送次数.vi" "小时数据发送次数"(w402) -> ()
                }
                frame True {
                  n249 = global read "全局 小时数据发送次数.vi" "小时数据发送次数"() -> (w406:i32)
                  n250 = Increment(x=w406) -> (x+1=w405:i32)
                  n251 = global write "全局 小时数据发送次数.vi" "小时数据发送次数"(w405) -> ()
                }
              }
            }
            frame "返回执行结果" {
            }
          }
        }
        frame "核查数据" {
          n252 = global read "全局1.vi" "枚举"() -> (w411:enum16{"返回请求应答", "上传数据", "返回执行结果"})
          n253 = case shown="\"上传数据\"" w411 {
            tunnel: ["QnRtn=1" w422 "ExeRtn=1"] -> w412
            tunnel: w410 -> [_ w415 _]
            tunnel: w409 -> [_ w414 _]
            frame "返回请求应答", Default {
            }
            frame "上传数据" {
              # "将非空数组的时间戳写入"
              n254 = call "数据发送组合-20200825 (子VI).vi"("枚举"=T4."核查数据", "插值后的数组元素"=w415) -> ("字符串"=w416:string)  [unwired: 9 in]
              n255 = global read "全局 小时数据发送次数.vi" "小时数据发送次数"() -> (w418:i32)
              n256 = Index Array(array=w414, index (row)=w418) -> (element=w421:string[])  [unwired: 1 in]
              n257 = Index Array(array=w421, index=0 ("索引")) -> (element=w420:string)
              n258 = call "规范分钟数据时间戳.vi"("字符串"=w420) -> ("result string"=w419:string)  [unwired: 10 in]
              n259 = Empty String/Path?(string/path=w419) -> (empty?=w424:bool)
              n260 = Format Into String(format string="DataTime=%s;%s" ("格式字符串"), w419, w416) -> (resulting string=w423:string)  [unwired: 2 in, 1 out]
              n261 = case shown="假" w424 {
                tunnel: [w427 ""] -> w422
                tunnel: w423 -> [w427 _]
                frame False {
                }
                frame True {
                }
              }
            }
            frame "返回执行结果" {
            }
          }
        }
        frame "空白测试", "跨度核查" {
          n262 = global read "全局1.vi" "枚举"() -> (w432:enum16{"返回请求应答", "上传数据", "返回执行结果"})
          n263 = case shown="\"上传数据\"" w432 {
            tunnel: ["QnRtn=1" w443 "ExeRtn=1"] -> w433
            tunnel: w431 -> [_ w437 _]
            tunnel: w430 -> [_ w435 _]
            frame "返回请求应答", Default {
            }
            frame "上传数据" {
              n264 = global read "全局 小时数据发送次数.vi" "小时数据发送次数"() -> (w441:i32)
              n265 = call "数据发送组合-20200825 (子VI).vi"("枚举"=T4."空白零点跨度数据", "插值后的数组元素"=w437) -> ("字符串"=w436:string)  [unwired: 9 in]
              n266 = Index Array(array=w435, index (row)=w441) -> (element=w447:string[])  [unwired: 1 in]
              n267 = Index Array(array=w447, index #1=0 ("索引"), index #2=3 ("索引"), index #3=7 ("索引")) -> (element #1=w440:string)  [unwired: 2 out]
              n268 = call "规范小时时间戳.vi"("字符串"=w440) -> ("result string"=w439:string)  [unwired: 10 in]
              n269 = Empty String/Path?(string/path=w439) -> (empty?=w444:bool)
              n270 = Format Into String(format string="DataTime=%s;%s" ("格式字符串"), w439, w436) -> (resulting string=w442:string)  [unwired: 2 in, 1 out]
              n271 = case shown="假" w444 {
                tunnel: [w450 ""] -> w443
                tunnel: w442 -> [w450 _]
                frame False {
                }
                frame True {
                }
              }
            }
            frame "返回执行结果" {
            }
          }
        }
      }
    }
    frame "小时数据" {
      # "发送小时数据"
      n272 = global read "全局1.vi" "枚举"() -> (w456:enum16{"返回请求应答", "上传数据", "返回执行结果"})
      n273 = case shown="\"上传数据\"" w456 {
        tunnel: ["QnRtn=1" w478 "ExeRtn=1"] -> w454
        tunnel: w455 -> [_ w466 _]
        tunnel: w453 -> [_ w463 _]
        frame "返回请求应答", Default {
          (unwired) 0 ("当前包数")
          n274 = global read "全局 数据数组大小.vi" "数据数组大小"() -> (w457:i32)
          n275 = global write "全局1.vi" "枚举"(enum16{"返回请求应答", "上传数据", "返回执行结果"}."上传数据" ("枚举")) -> ()
          n276 = Equal To 0?(x=w457) -> (x = 0?=w458:bool)
          n277 = case shown="真" w458 {
            frame False {
            }
            frame True {
              n278 = global read "全局 小时数据发送次数.vi" "小时数据发送次数"() -> (w462:i32)
              n279 = Increment(x=w462) -> (x+1=w461:i32)
              n280 = global write "全局 小时数据发送次数.vi" "小时数据发送次数"(w461) -> ()
            }
          }
        }
        frame "上传数据" {
          n281 = call "数据发送组合-20200825 (子VI).vi"("枚举"=enum16{"小时数据", "实时数据"}."小时数据", "插值后的数组元素"=w466) -> ("字符串"=w464:string)  [unwired: 9 in]
          n282 = global read "全局 小时数据发送次数.vi" "小时数据发送次数"() -> (w477:i32)
          n283 = Empty String/Path?(string/path=w464) -> (empty?=w479:bool)
          n284 = Index Array(array=w463, index (row)=w477) -> (element=w476:string[])  [unwired: 1 in]
          n285 = Index Array(array=w476, index=0 ("索引")) -> (element=w474:string)
          n286 = call "规范小时时间戳.vi"("字符串"=w474) -> ("result string"=w471:string)  [unwired: 10 in]
          n287 = Format Into String(format string="DataTime=%s;", w471) -> (resulting string=w473:string)  [unwired: 2 in, 1 out]
          n288 = Concatenate Strings(w473, w464) -> (w468:string)
          n289 = String Length(string=w468) -> (length=w470:i32)
          n290 = Decrement(x=w470) -> (x-1=w469:i32)
          n291 = String Subset(string=w468, length (rest)=w469) -> (substring=w467:string)  [unwired: 1 in]
          n292 = case shown="假" w479 {
            tunnel: [w480 ""] -> w478
            tunnel: w467 -> [w480 _]
            frame False {
            }
            frame True {
            }
          }
        }
        frame "返回执行结果" {
          (unwired) 0 ("当前包数")
          n293 = global write "全局1.vi" "枚举"(enum16{"返回请求应答", "上传数据", "返回执行结果"}."返回请求应答" ("枚举")) -> ()
        }
      }
    }
    frame "剖面数据" {
      # "{\"data\":[{\"time\":\"21-06-08 01:08:00\",\"w01010Value\":23,\"w01001Value\":7,\"w01009Value\":6,\"w01014Value\":22,\"w01003Value\":100,\"depth\":0.5,\"row\":3},{\"time\":\"21-06-08 01:08:00\",\"w01010Value\":22,\"w01001Value\":8,\"w01009Value\":7,\"w01014Value\":25,\"w01003Value\":96,\"depth\":0.8,\"row\":3},{\"time\":\"21-06-08 01:08:00\",\"w01010Value\":21,\"w01001Value\":7,\"w01009Value\":7,\"w01014Value\":24,\"w01003Value\":95,\"depth\":1,\"row\":3}]}"
      # "发送剖面数据"
      n294 = global read "全局1.vi" "枚举"() -> (w484:enum16{"返回请求应答", "上传数据", "返回执行结果"})
      n295 = case shown="\"上传数据\"" w484 {
        tunnel: ["QnRtn=1" w495 "ExeRtn=1"] -> w485
        frame "返回请求应答", Default {
          (unwired) 0 ("当前包数")
          n296 = global read "全局 数据数组大小.vi" "数据数组大小"() -> (w486:i32)
          n297 = global write "全局1.vi" "枚举"(enum16{"返回请求应答", "上传数据", "返回执行结果"}."上传数据" ("枚举")) -> ()
          n298 = Equal To 0?(x=w486) -> (x = 0?=w487:bool)
          n299 = case shown="真" w487 {
            frame False {
            }
            frame True {
              n300 = global read "全局 小时数据发送次数.vi" "小时数据发送次数"() -> (w491:i32)
              n301 = Increment(x=w491) -> (x+1=w490:i32)
              n302 = global write "全局 小时数据发送次数.vi" "小时数据发送次数"(w490) -> ()
            }
          }
        }
        frame "上传数据" {
          n303 = global read "断电保存全局.vi" "数据发送协议"() -> (w494:enum16{"2005-212协议", "2017-212协议"})
          n304 = case shown="\"2017-212协议\", 默认" w494 {
            tunnel: ["" ("编码输出") w516] -> w493
            tunnel: [_ w512] -> w492
            frame "2005-212协议" {
            }
            frame "2017-212协议", Default {
              w506 = 0 ("索引 (行)")
              (unwired) "w01010" ("污染物编码")
              (unwired) "w01016" ("污染物编码")
              (unwired) "w01003" ("污染物编码")
              (unwired) "w01014" ("污染物编码")
              # "时间,测量模式,数据类型,数据标识,层数,Temp,SpCond,Cond,Sal,TDS,pH,pHmV,ORP,ODO%,ODOmg/L,Turb,Chla,Depth,"
              n305 = global read "全局 小时数据发送次数.vi" "小时数据发送次数"() -> (w515:i32)
              n306 = global read "全局 所有参数.vi" "剖面多参数"() -> (w503:string[][])
              n307 = global read "全局 数据数组大小.vi" "分包标准"() -> (w514:i32)
              n308 = global read "全局 所有参数.vi" "columns"() -> (w513:string[])
              n309 = Array Subset(array=w503, index (row)=w515, length (row)=w514) -> (w512:string[][])  [unwired: 2 in]
              n310 = Array Subset(array=w503, index (row)=0 ("索引"), length (row)=1 ("长度")) -> (w501:string[][])  [unwired: 2 in]
              n311 = call "新剖面数据组合.vi"("columns"=w513, "剖面数据"=w512) -> ("结果字符串"=w510:string)  [unwired: 9 in]
              n312 = Index Array(array=w501, index (row) #1=w506, index (col) #1=0 ("索引 (行)"), index (row) #2=w506, index (col) #2=1 ("索引 (列)"), index (row) #3=w506, index (col) #3=2 ("索引 (列)")) -> (element #1=w499:string, element #2=w505:string, element #3=w504:string)
              n313 = call "规范分钟数据时间戳.vi"("字符串"=w499) -> ("result string"=w498:string)  [unwired: 10 in]
              n314 = Format Into String(format string="DataTime=%s;total=%s;waterdepth=%s;data=%s", w498, w505, w504, w510) -> (resulting string=w509:string)  [unwired: 2 in, 1 out]
              n315 = Empty String/Path?(string/path=w510) -> (empty?=w517:bool)
              n316 = case shown="真" w517 {
                tunnel: [w519 ""] -> w516
                tunnel: w509 -> [w519 _]
                frame False {
                }
                frame True {
                }
              }
            }
          }
          n317 = Empty String/Path?(string/path=w493) -> (empty?=w496:bool)
          n318 = case shown="假" w496 {
            tunnel: [w526 ""] -> w495
            tunnel: w493 -> [w526 _]
            tunnel: w492 -> [w525 w527]
            frame False {
              n319 = global read "全局 小时数据发送次数.vi" "小时数据发送次数"() -> (w522:i32)
              n320 = Array Size(array=w525) -> (size(s)=w524:i32[])
              n321 = Index Array(array=w524) -> (element=w523:i32)  [unwired: 1 in]
              n322 = Add(x=w523, y=w522) -> (x+y=w521:i32)
              n323 = global write "全局 小时数据发送次数.vi" "小时数据发送次数"(w521) -> ()
            }
            frame True {
              n324 = global read "全局 小时数据发送次数.vi" "小时数据发送次数"() -> (w529:i32)
              n325 = Array Size(array=w527) -> (size(s)=w531:i32[])
              n326 = Index Array(array=w531) -> (element=w530:i32)  [unwired: 1 in]
              n327 = Add(x=w530, y=w529) -> (x+y=w528:i32)
              n328 = global write "全局 小时数据发送次数.vi" "小时数据发送次数"(w528) -> ()
            }
          }
        }
        frame "返回执行结果" {
          (unwired) 0 ("当前包数")
          n329 = global write "全局1.vi" "枚举"(enum16{"返回请求应答", "上传数据", "返回执行结果"}."返回请求应答" ("枚举")) -> ()
        }
      }
    }
    frame "剖面多参数H" {
      # "发送小时数据"
      n330 = global read "全局1.vi" "枚举"() -> (w535:enum16{"返回请求应答", "上传数据", "返回执行结果"})
      n331 = case shown="\"上传数据\"" w535 {
        tunnel: ["QnRtn=1" w545 "ExeRtn=1"] -> w536
        frame "返回请求应答", Default {
          (unwired) 0 ("当前包数")
          n332 = global read "全局 数据数组大小.vi" "数据数组大小"() -> (w537:i32)
          n333 = global write "全局1.vi" "枚举"(enum16{"返回请求应答", "上传数据", "返回执行结果"}."上传数据" ("枚举")) -> ()
          n334 = Equal To 0?(x=w537) -> (x = 0?=w538:bool)
          n335 = case shown="真" w538 {
            frame False {
            }
            frame True {
              n336 = global read "全局 小时数据发送次数.vi" "小时数据发送次数"() -> (w542:i32)
              n337 = Increment(x=w542) -> (x+1=w541:i32)
              n338 = global write "全局 小时数据发送次数.vi" "小时数据发送次数"(w541) -> ()
            }
          }
        }
        frame "上传数据" {
          n339 = global read "断电保存全局.vi" "数据发送协议"() -> (w544:enum16{"2005-212协议", "2017-212协议"})
          n340 = case shown="\"2017-212协议\", 默认" w544 {
            tunnel: ["" ("编码输出") w550] -> w543
            frame "2005-212协议" {
            }
            frame "2017-212协议", Default {
              (unwired) "w01010" ("污染物编码")
              (unwired) "w01016" ("污染物编码")
              (unwired) "w01003" ("污染物编码")
              (unwired) "w01009" ("污染物编码")
              (unwired) "w01001" ("污染物编码")
              (unwired) "w01014" ("污染物编码")
              (unwired) "w01100" ("污染物编码")
              # "时间,测量模式,数据类型,数据标识,层数,Temp,SpCond,Cond,Sal,TDS,pH,pHmV,ORP,ODO%,ODOmg/L,Turb,Chla,Depth,"
              n341 = global read "全局 小时数据发送次数.vi" "小时数据发送次数"() -> (w568:i32)
              n342 = global read "全局 所有参数.vi" "剖面多参数"() -> (w571:string[][])
              n343 = Index Array(array=w571, index (row)=w568) -> (element=w569:string[])  [unwired: 1 in]
              n344 = Index Array(array=w569, index #1=0 ("索引")) -> (element #1=w553:string, element #3=w567:string, element #4=w566:string, element #5=w565:string, element #6=w564:string, element #7=w563:string, element #11=w561:string, element #13=w560:string, element #15=w559:string, element #16=w558:string, element #17=w557:string)  [unwired: 16 in, 6 out]
              n345 = call "规范小时时间戳.vi"("字符串"=w553) -> ("result string"=w554:string)  [unwired: 10 in]
              n346 = Build Array(w564, w563, w561, w560, w559, w558, w557) -> (w562:string[])
              n347 = call "剖面多参数组合(子VI).vi"("数据类型实时小时"="-Avg=", "数据值"=w562, "层数"=w565, "数据标识"=w566, "数据类型"=w567) -> ("编码输出"=w549:string)  [unwired: 6 in]
              n348 = Format Into String(format string="DataTime=%s;", w554) -> (resulting string=w555:string)  [unwired: 2 in, 1 out]
              n349 = Empty String/Path?(string/path=w549) -> (empty?=w552:bool)
              n350 = Concatenate Strings(w555, w549) -> (w551:string)
              n351 = case shown="真" w552 {
                tunnel: [w572 ""] -> w550
                tunnel: w551 -> [w572 _]
                frame False {
                }
                frame True {
                }
              }
            }
          }
          n352 = Empty String/Path?(string/path=w543) -> (empty?=w546:bool)
          n353 = case shown="假" w546 {
            tunnel: [w576 ""] -> w545
            tunnel: w543 -> [w576 _]
            frame False {
              n354 = global read "全局 小时数据发送次数.vi" "小时数据发送次数"() -> (w575:i32)
              n355 = Increment(x=w575) -> (x+1=w574:i32)
              n356 = global write "全局 小时数据发送次数.vi" "小时数据发送次数"(w574) -> ()
            }
            frame True {
              n357 = global read "全局 小时数据发送次数.vi" "小时数据发送次数"() -> (w578:i32)
              n358 = Increment(x=w578) -> (x+1=w577:i32)
              n359 = global write "全局 小时数据发送次数.vi" "小时数据发送次数"(w577) -> ()
            }
          }
        }
        frame "返回执行结果" {
          (unwired) 0 ("当前包数")
          n360 = global write "全局1.vi" "枚举"(enum16{"返回请求应答", "上传数据", "返回执行结果"}."返回请求应答" ("枚举")) -> ()
        }
      }
    }
    frame "剖面多参数S" {
      # "发送实时数据"
      n361 = global read "全局1.vi" "枚举"() -> (w582:enum16{"返回请求应答", "上传数据", "返回执行结果"})
      n362 = case shown="\"上传数据\"" w582 {
        tunnel: ["QnRtn=1" w592 "ExeRtn=1"] -> w583
        frame "返回请求应答", Default {
          (unwired) 0 ("当前包数")
          n363 = global read "全局 数据数组大小.vi" "数据数组大小"() -> (w584:i32)
          n364 = global write "全局1.vi" "枚举"(enum16{"返回请求应答", "上传数据", "返回执行结果"}."上传数据" ("枚举")) -> ()
          n365 = Equal To 0?(x=w584) -> (x = 0?=w585:bool)
          n366 = case shown="真" w585 {
            frame False {
            }
            frame True {
              n367 = global read "全局 小时数据发送次数.vi" "小时数据发送次数"() -> (w589:i32)
              n368 = Increment(x=w589) -> (x+1=w588:i32)
              n369 = global write "全局 小时数据发送次数.vi" "小时数据发送次数"(w588) -> ()
            }
          }
        }
        frame "上传数据" {
          n370 = global read "断电保存全局.vi" "数据发送协议"() -> (w591:enum16{"2005-212协议", "2017-212协议"})
          n371 = case shown="\"2017-212协议\", 默认" w591 {
            tunnel: ["" ("编码输出") w599] -> w590
            frame "2005-212协议" {
            }
            frame "2017-212协议", Default {
              (unwired) "w01010" ("污染物编码")
              (unwired) "w01016" ("污染物编码")
              (unwired) "w01003" ("污染物编码")
              (unwired) "w01009" ("污染物编码")
              (unwired) "w01001" ("污染物编码")
              (unwired) "w01014" ("污染物编码")
              (unwired) "w01100" ("污染物编码")
              # "时间,测量模式,数据类型,数据标识,层数,Temp,SpCond,Cond,Sal,TDS,pH,pHmV,ORP,ODO%,ODOmg/L,Turb,Chla,Depth,"
              n372 = global read "全局 小时数据发送次数.vi" "小时数据发送次数"() -> (w615:i32)
              n373 = global read "全局 所有参数.vi" "剖面多参数"() -> (w618:string[][])
              n374 = Index Array(array=w618, index (row)=w615) -> (element=w616:string[])  [unwired: 1 in]
              n375 = Index Array(array=w616, index #1=0 ("索引")) -> (element #1=w596:string, element #3=w614:string, element #4=w613:string, element #5=w612:string, element #6=w611:string, element #7=w610:string, element #11=w608:string, element #13=w607:string, element #15=w606:string, element #16=w605:string, element #17=w604:string)  [unwired: 16 in, 6 out]
              n376 = call "规范时间戳.vi"("字符串"=w596) -> ("result string"=w595:string)  [unwired: 10 in]
              n377 = Build Array(w611, w610, w608, w607, w606, w605, w604) -> (w609:string[])
              n378 = call "剖面多参数组合(子VI).vi"("数据类型实时小时"="-Rtd=", "数据值"=w609, "层数"=w612, "数据标识"=w613, "数据类型"=w614) -> ("编码输出"=w598:string)  [unwired: 6 in]
              n379 = Format Into String(format string="DataTime=%s;", w595) -> (resulting string=w602:string)  [unwired: 2 in, 1 out]
              n380 = Empty String/Path?(string/path=w598) -> (empty?=w601:bool)
              n381 = Concatenate Strings(w602, w598) -> (w600:string)
              n382 = case shown="假" w601 {
                tunnel: [w619 ""] -> w599
                tunnel: w600 -> [w619 _]
                frame False {
                }
                frame True {
                }
              }
            }
          }
          n383 = Empty String/Path?(string/path=w590) -> (empty?=w593:bool)
          n384 = case shown="假" w593 {
            tunnel: [w623 ""] -> w592
            tunnel: w590 -> [w623 _]
            frame False {
              n385 = global read "全局 小时数据发送次数.vi" "小时数据发送次数"() -> (w622:i32)
              n386 = Increment(x=w622) -> (x+1=w621:i32)
              n387 = global write "全局 小时数据发送次数.vi" "小时数据发送次数"(w621) -> ()
            }
            frame True {
              n388 = global read "全局 小时数据发送次数.vi" "小时数据发送次数"() -> (w625:i32)
              n389 = Increment(x=w625) -> (x+1=w624:i32)
              n390 = global write "全局 小时数据发送次数.vi" "小时数据发送次数"(w624) -> ()
            }
          }
        }
        frame "返回执行结果" {
          (unwired) 0 ("当前包数")
          n391 = global write "全局1.vi" "枚举"(enum16{"返回请求应答", "上传数据", "返回执行结果"}."返回请求应答" ("枚举")) -> ()
        }
      }
    }
    frame "提取小时数据" {
      # "发送小时数据"
      n392 = global read "全局 小时数据发送次数.vi" "小时数据发送次数"() -> (w631:i32)
      n393 = Index Array(array=w633, index (row)=w631) -> (element=w630:string[])  [unwired: 1 in]
      n394 = global read "全局1.vi" "枚举"() -> (w632:enum16{"返回请求应答", "上传数据", "返回执行结果"})
      n395 = case shown="\"上传数据\"" w632 {
        tunnel: ["QnRtn=1" w648 "ExeRtn=1"] -> w634
        tunnel: w630 -> [_ w650 _]
        tunnel: w629 -> [_ w640 _]
        frame "返回请求应答", Default {
          n396 = global read "全局 数据数组大小.vi" "数据数组大小"() -> (w635:i32)
          n397 = Equal To 0?(x=w635) -> (x = 0?=w636:bool)
          n398 = case shown="真" w636 {
            frame False {
            }
            frame True {
              n399 = global read "全局 小时数据发送次数.vi" "小时数据发送次数"() -> (w639:i32)
              n400 = Increment(x=w639) -> (x+1=w638:i32)
              n401 = global write "全局 小时数据发送次数.vi" "小时数据发送次数"(w638) -> ()
            }
          }
        }
        frame "上传数据" {
          n402 = Index Array(array=w650, index #2=1 ("索引")) -> (element #1=w643:string)  [unwired: 1 in, 1 out]
          n403 = call "规范小时时间戳.vi"("字符串"=w643) -> ("result string"=w644:string)  [unwired: 10 in]
          n404 = call "数据发送组合-20200825 (子VI).vi"("枚举"=T4."提取小时数据", "插值后的数组元素"=w640) -> ("字符串"=w641:string)  [unwired: 9 in]
          n405 = Format Into String(format string="DataTime=%s;", w644) -> (resulting string=w647:string)  [unwired: 2 in, 1 out]
          n406 = Empty String/Path?(string/path=w641) -> (empty?=w649:bool)
          n407 = Concatenate Strings(w647, w641) -> (w645:string)
          n408 = case shown="假" w649 {
            tunnel: [w654 ""] -> w648
            tunnel: w645 -> [w654 _]
            frame False {
              n409 = global read "全局 小时数据发送次数.vi" "小时数据发送次数"() -> (w653:i32)
              n410 = Increment(x=w653) -> (x+1=w652:i32)
              n411 = global write "全局 小时数据发送次数.vi" "小时数据发送次数"(w652) -> ()
            }
            frame True {
              n412 = global read "全局 小时数据发送次数.vi" "小时数据发送次数"() -> (w656:i32)
              n413 = Increment(x=w656) -> (x+1=w655:i32)
              n414 = global write "全局 小时数据发送次数.vi" "小时数据发送次数"(w655) -> ()
            }
          }
        }
        frame "返回执行结果" {
        }
      }
    }
    frame "提取实时数据" {
      # "提取实时数据"
      n415 = global read "全局 小时数据发送次数.vi" "小时数据发送次数"() -> (w661:i32)
      n416 = Index Array(array=w664, index (row)=w661) -> (element=w660:string[])  [unwired: 1 in]
      n417 = global read "全局1.vi" "枚举"() -> (w662:enum16{"返回请求应答", "上传数据", "返回执行结果"})
      n418 = case shown="\"上传数据\"" w662 {
        tunnel: ["QnRtn=1" w673 "ExeRtn=1"] -> w663
        tunnel: w660 -> [_ w679 _]
        tunnel: w659 -> [_ w671 _]
        frame "返回请求应答", Default {
          n419 = global read "全局 数据数组大小.vi" "数据数组大小"() -> (w665:i32)
          n420 = Equal To 0?(x=w665) -> (x = 0?=w666:bool)
          n421 = case shown="真" w666 {
            frame False {
            }
            frame True {
              n422 = global read "全局 小时数据发送次数.vi" "小时数据发送次数"() -> (w669:i32)
              n423 = Increment(x=w669) -> (x+1=w668:i32)
              n424 = global write "全局 小时数据发送次数.vi" "小时数据发送次数"(w668) -> ()
            }
          }
        }
        frame "上传数据" {
          n425 = Index Array(array=w679, index #1=0 ("索引"), index #2=3 ("索引"), index #3=5 ("索引")) -> (element #1=w677:string)  [unwired: 2 out]
          n426 = call "规范时间戳.vi"("字符串"=w677) -> ("result string"=w676:string)  [unwired: 10 in]
          n427 = call "数据发送组合-20200825 (子VI).vi"("枚举"=T4."提取实时数据", "插值后的数组元素"=w671) -> ("字符串"=w670:string)  [unwired: 9 in]
          n428 = Empty String/Path?(string/path=w676) -> (empty?=w675:bool)
          n429 = Format Into String(format string="DataTime=%s;%s" ("格式字符串"), w676, w670) -> (resulting string=w674:string)  [unwired: 2 in, 1 out]
          n430 = case shown="真" w675 {
            tunnel: [w683 ""] -> w673
            tunnel: w674 -> [w683 _]
            frame False {
              n431 = global read "全局 小时数据发送次数.vi" "小时数据发送次数"() -> (w685:i32)
              n432 = Increment(x=w685) -> (x+1=w684:i32)
              n433 = global write "全局 小时数据发送次数.vi" "小时数据发送次数"(w684) -> ()
            }
            frame True {
              n434 = global read "全局 小时数据发送次数.vi" "小时数据发送次数"() -> (w687:i32)
              n435 = Increment(x=w687) -> (x+1=w686:i32)
              n436 = global write "全局 小时数据发送次数.vi" "小时数据发送次数"(w686) -> ()
            }
          }
        }
        frame "返回执行结果" {
        }
      }
    }
    frame "核查数据" {
      # "提取标样核查数据"
      n437 = global read "全局 小时数据发送次数.vi" "小时数据发送次数"() -> (w693:i32)
      n438 = Index Array(array=w690, index (row)=w693) -> (element=w692:string[])  [unwired: 1 in]
      n439 = global read "全局1.vi" "枚举"() -> (w694:enum16{"返回请求应答", "上传数据", "返回执行结果"})
      n440 = case shown="\"上传数据\"" w694 {
        tunnel: ["QnRtn=1" w706 "ExeRtn=1"] -> w695
        tunnel: w692 -> [_ w712 _]
        tunnel: w691 -> [_ w702 _]
        frame "返回请求应答", Default {
          n441 = global read "全局 数据数组大小.vi" "数据数组大小"() -> (w697:i32)
          n442 = Equal To 0?(x=w697) -> (x = 0?=w696:bool)
          n443 = case shown="真" w696 {
            frame False {
            }
            frame True {
              n444 = global read "全局 小时数据发送次数.vi" "小时数据发送次数"() -> (w700:i32)
              n445 = Increment(x=w700) -> (x+1=w699:i32)
              n446 = global write "全局 小时数据发送次数.vi" "小时数据发送次数"(w699) -> ()
            }
          }
        }
        frame "上传数据" {
          # "将非空数组的时间戳写入"
          n447 = Index Array(array=w712, index #1=0 ("索引"), index #2=3 ("索引"), index #3=6 ("索引")) -> (element #1=w705:string)  [unwired: 2 out]
          n448 = call "数据发送组合-20200825 (子VI).vi"("枚举"=T4."核查数据", "插值后的数组元素"=w702) -> ("字符串"=w701:string)  [unwired: 9 in]
          n449 = call "规范时间戳.vi"("字符串"=w705) -> ("result string"=w704:string)  [unwired: 10 in]
          n450 = Empty String/Path?(string/path=w704) -> (empty?=w708:bool)
          n451 = Format Into String(format string="DataTime=%s;%s" ("格式字符串"), w704, w701) -> (resulting string=w707:string)  [unwired: 2 in, 1 out]
          n452 = case shown="假" w708 {
            tunnel: [w716 ""] -> w706
            tunnel: w707 -> [w716 _]
            frame False {
              n453 = global read "全局 小时数据发送次数.vi" "小时数据发送次数"() -> (w715:i32)
              n454 = Increment(x=w715) -> (x+1=w714:i32)
              n455 = global write "全局 小时数据发送次数.vi" "小时数据发送次数"(w714) -> ()
            }
            frame True {
              n456 = global read "全局 小时数据发送次数.vi" "小时数据发送次数"() -> (w718:i32)
              n457 = Increment(x=w718) -> (x+1=w717:i32)
              n458 = global write "全局 小时数据发送次数.vi" "小时数据发送次数"(w717) -> ()
            }
          }
        }
        frame "返回执行结果" {
        }
      }
    }
    frame "空白测试", "跨度核查", "零点核查" {
      # "提取空白测试数据/零点核查数据/跨度核查数据"
      n459 = global read "全局 小时数据发送次数.vi" "小时数据发送次数"() -> (w724:i32)
      n460 = Index Array(array=w721, index (row)=w724) -> (element=w723:string[])  [unwired: 1 in]
      n461 = global read "全局1.vi" "枚举"() -> (w725:enum16{"返回请求应答", "上传数据", "返回执行结果"})
      n462 = case shown="\"上传数据\"" w725 {
        tunnel: ["QnRtn=1" w737 "ExeRtn=1"] -> w726
        tunnel: w723 -> [_ w742 _]
        tunnel: w722 -> [_ w733 _]
        frame "返回请求应答", Default {
          (unwired) 0 ("当前包数")
          n463 = global read "全局 数据数组大小.vi" "数据数组大小"() -> (w728:i32)
          n464 = Equal To 0?(x=w728) -> (x = 0?=w727:bool)
          n465 = case shown="真" w727 {
            frame False {
            }
            frame True {
              n466 = global read "全局 小时数据发送次数.vi" "小时数据发送次数"() -> (w731:i32)
              n467 = Increment(x=w731) -> (x+1=w730:i32)
              n468 = global write "全局 小时数据发送次数.vi" "小时数据发送次数"(w730) -> ()
            }
          }
        }
        frame "上传数据" {
          # "将非空数组的时间戳写入"
          n469 = Index Array(array=w742, index #1=0 ("索引"), index #2=3 ("索引")) -> (element #1=w736:string)  [unwired: 1 out]
          n470 = call "数据发送组合-20200825 (子VI).vi"("枚举"=T4."空白零点跨度数据", "插值后的数组元素"=w733) -> ("字符串"=w732:string)  [unwired: 9 in]
          n471 = call "规范时间戳.vi"("字符串"=w736) -> ("result string"=w735:string)  [unwired: 10 in]
          n472 = Empty String/Path?(string/path=w735) -> (empty?=w739:bool)
          n473 = Format Into String(format string="DataTime=%s;%s" ("格式字符串"), w735, w732) -> (resulting string=w738:string)  [unwired: 2 in, 1 out]
          n474 = case shown="假" w739 {
            tunnel: [w746 ""] -> w737
            tunnel: w738 -> [w746 _]
            frame False {
              n475 = global read "全局 小时数据发送次数.vi" "小时数据发送次数"() -> (w745:i32)
              n476 = Increment(x=w745) -> (x+1=w744:i32)
              n477 = global write "全局 小时数据发送次数.vi" "小时数据发送次数"(w744) -> ()
            }
            frame True {
              n478 = global read "全局 小时数据发送次数.vi" "小时数据发送次数"() -> (w748:i32)
              n479 = Increment(x=w748) -> (x+1=w747:i32)
              n480 = global write "全局 小时数据发送次数.vi" "小时数据发送次数"(w747) -> ()
            }
          }
        }
        frame "返回执行结果" {
        }
      }
    }
    frame "提取加标回收" {
      # "提取加标回收数据"
      n481 = global read "全局1.vi" "枚举"() -> (w754:enum16{"返回请求应答", "上传数据", "返回执行结果"})
      n482 = case shown="\"上传数据\"" w754 {
        tunnel: ["QnRtn=1" w766 "ExeRtn=1"] -> w752
        tunnel: w753 -> [_ w768 _]
        tunnel: w751 -> [_ w760 _]
        frame "返回请求应答", Default {
          n483 = global read "全局 数据数组大小.vi" "数据数组大小"() -> (w755:i32)
          n484 = Equal To 0?(x=w755) -> (x = 0?=w756:bool)
          n485 = case shown="真" w756 {
            frame False {
            }
            frame True {
              n486 = global read "全局 小时数据发送次数.vi" "小时数据发送次数"() -> (w759:i32)
              n487 = Increment(x=w759) -> (x+1=w758:i32)
              n488 = global write "全局 小时数据发送次数.vi" "小时数据发送次数"(w758) -> ()
            }
          }
        }
        frame "上传数据" {
          # "w01001-Check=63.0,w01001-WaterTime=20160801080000,w01001-Water=45.23,w01001-Chroma=1000,w01001-Volume=0.2,w01001-DVolume=200,w01003-Flag=N;"
          # "CODMn"
          n489 = global read "全局 小时数据发送次数.vi" "小时数据发送次数"() -> (w763:i32)
          n490 = call "数据发送组合-20200825 (子VI).vi"("枚举"=T4."加标回收测试", "插值后的数组元素"=w760) -> ("字符串"=w761:string)  [unwired: 9 in]
          n491 = call "加标回收数据组合 (子VI).vi"("小时数据发送次数"=w763, "数据"=w768, "污染物编码"="w01019") -> ("datatime"=w770:string)  [unwired: 7 in, 1 out]
          n492 = call "规范时间戳.vi"("字符串"=w770) -> ("result string"=w769:string)  [unwired: 10 in]
          n493 = Empty String/Path?(string/path=w769) -> (empty?=w765:bool)
          n494 = Format Into String(format string="DataTime=%s;%s" ("格式字符串"), w769, w761) -> (resulting string=w767:string)  [unwired: 2 in, 1 out]
          n495 = case shown="真" w765 {
            tunnel: [w774 ""] -> w766
            tunnel: w767 -> [w774 _]
            frame False {
              n496 = global read "全局 小时数据发送次数.vi" "小时数据发送次数"() -> (w773:i32)
              n497 = Increment(x=w773) -> (x+1=w772:i32)
              n498 = global write "全局 小时数据发送次数.vi" "小时数据发送次数"(w772) -> ()
            }
            frame True {
              n499 = global read "全局 小时数据发送次数.vi" "小时数据发送次数"() -> (w776:i32)
              n500 = Increment(x=w776) -> (x+1=w775:i32)
              n501 = global write "全局 小时数据发送次数.vi" "小时数据发送次数"(w775) -> ()
            }
          }
        }
        frame "返回执行结果" {
        }
      }
    }
    frame "提取平行样" {
      # "提取平行样数据"
      n502 = global read "全局1.vi" "枚举"() -> (w782:enum16{"返回请求应答", "上传数据", "返回执行结果"})
      n503 = case shown="\"上传数据\"" w782 {
        tunnel: ["QnRtn=1" w798 "ExeRtn=1"] -> w781
        tunnel: w780 -> [_ w792 _]
        tunnel: w779 -> [_ w788 _]
        frame "返回请求应答", Default {
          n504 = global read "全局 数据数组大小.vi" "数据数组大小"() -> (w783:i32)
          n505 = Equal To 0?(x=w783) -> (x = 0?=w784:bool)
          n506 = case shown="真" w784 {
            frame False {
            }
            frame True {
              n507 = global read "全局 小时数据发送次数.vi" "小时数据发送次数"() -> (w787:i32)
              n508 = Increment(x=w787) -> (x+1=w786:i32)
              n509 = global write "全局 小时数据发送次数.vi" "小时数据发送次数"(w786) -> ()
            }
          }
        }
        frame "上传数据" {
          # "CODMn"
          n510 = global read "全局 小时数据发送次数.vi" "小时数据发送次数"() -> (w791:i32)
          n511 = call "数据发送组合-20200825 (子VI).vi"("枚举"=T4."平行样测试", "插值后的数组元素"=w788) -> ("字符串"=w789:string)  [unwired: 9 in]
          n512 = Index Array(array=w792, index (row)=w791) -> (element=w796:string[])  [unwired: 1 in]
          n513 = Index Array(array=w796, index=0 ("索引")) -> (element=w793:string)
          n514 = call "规范时间戳.vi"("字符串"=w793) -> ("result string"=w794:string)  [unwired: 10 in]
          n515 = Empty String/Path?(string/path=w793) -> (empty?=w797:bool)
          n516 = Format Into String(format string="DataTime=%s;%s" ("格式字符串"), w794, w789) -> (resulting string=w799:string)  [unwired: 2 in, 1 out]
          n517 = case shown="真" w797 {
            tunnel: [w803 ""] -> w798
            tunnel: w799 -> [w803 _]
            frame False {
              n518 = global read "全局 小时数据发送次数.vi" "小时数据发送次数"() -> (w802:i32)
              n519 = Increment(x=w802) -> (x+1=w801:i32)
              n520 = global write "全局 小时数据发送次数.vi" "小时数据发送次数"(w801) -> ()
            }
            frame True {
              n521 = global read "全局 小时数据发送次数.vi" "小时数据发送次数"() -> (w805:i32)
              n522 = Increment(x=w805) -> (x+1=w804:i32)
              n523 = global write "全局 小时数据发送次数.vi" "小时数据发送次数"(w804) -> ()
            }
          }
        }
        frame "返回执行结果" {
        }
      }
    }
    frame "提取集成干预" {
      # "提取平行样数据"
      n524 = global read "全局1.vi" "枚举"() -> (w811:enum16{"返回请求应答", "上传数据", "返回执行结果"})
      n525 = case shown="\"上传数据\"" w811 {
        tunnel: ["QnRtn=1" w828 "ExeRtn=1"] -> w810
        tunnel: w809 -> [_ w823 _]
        tunnel: w808 -> [_ w820 _]
        frame "返回请求应答", Default {
          n526 = global read "全局 数据数组大小.vi" "数据数组大小"() -> (w812:i32)
          n527 = Equal To 0?(x=w812) -> (x = 0?=w813:bool)
          n528 = case shown="真" w813 {
            frame False {
            }
            frame True {
              n529 = global read "全局 小时数据发送次数.vi" "小时数据发送次数"() -> (w816:i32)
              n530 = Increment(x=w816) -> (x+1=w815:i32)
              n531 = global write "全局 小时数据发送次数.vi" "小时数据发送次数"(w815) -> ()
            }
          }
        }
        frame "上传数据" {
          # "CODMn"
          n532 = global read "全局 小时数据发送次数.vi" "小时数据发送次数"() -> (w824:i32)
          n533 = call "数据发送组合-20200825 (子VI).vi"("枚举"=T4."集成干预测试", "插值后的数组元素"=w820) -> ("字符串"=w821:string)  [unwired: 9 in]
          n534 = Index Array(array=w823, index (row)=w824) -> (element=w826:string[])  [unwired: 1 in]
          n535 = global read "断电保存全局.vi" "应用环境"() -> (w819:enum16{"STD", "GB212"})
          n536 = Index Array(array=w826, index=0 ("索引")) -> (element=w818:string)
          n537 = case shown="\"STD\", 默认" w819 {
            tunnel: [w832 w833] -> w817
            tunnel: w818 -> [w831 w834]
            frame "STD", Default {
              n538 = call "规范时间戳.vi"("字符串"=w831) -> ("result string"=w832:string)  [unwired: 10 in]
            }
            frame "GB212" {
              n539 = call "规范分钟数据时间戳.vi"("字符串"=w834) -> ("result string"=w833:string)  [unwired: 10 in]
            }
          }
          n540 = Empty String/Path?(string/path=w818) -> (empty?=w827:bool)
          n541 = Format Into String(format string="DataTime=%s;%s" ("格式字符串"), w817, w821) -> (resulting string=w829:string)  [unwired: 2 in, 1 out]
          n542 = case shown="真" w827 {
            tunnel: [w837 ""] -> w828
            tunnel: w829 -> [w837 _]
            frame False {
              n543 = global read "全局 小时数据发送次数.vi" "小时数据发送次数"() -> (w836:i32)
              n544 = Increment(x=w836) -> (x+1=w835:i32)
              n545 = global write "全局 小时数据发送次数.vi" "小时数据发送次数"(w835) -> ()
            }
            frame True {
              n546 = global read "全局 小时数据发送次数.vi" "小时数据发送次数"() -> (w839:i32)
              n547 = Increment(x=w839) -> (x+1=w838:i32)
              n548 = global write "全局 小时数据发送次数.vi" "小时数据发送次数"(w838) -> ()
            }
          }
        }
        frame "返回执行结果" {
        }
      }
    }
    frame "操作日志" {
      n549 = global read "全局 小时数据发送次数.vi" "小时数据发送次数"() -> (w844:i32)
      n550 = Index Array(array=w846, index (row)=w844) -> (element=w843:string[])  [unwired: 1 in]
      n551 = global read "全局1.vi" "枚举"() -> (w845:enum16{"返回请求应答", "上传数据", "返回执行结果"})
      n552 = case shown="\"上传数据\"" w845 {
        tunnel: ["QnRtn=1" w864 "ExeRtn=1"] -> w847
        tunnel: w843 -> [_ w866 _]
        tunnel: w842 -> [_ w854 _]
        frame "返回请求应答", Default {
          n553 = global read "全局 数据数组大小.vi" "数据数组大小"() -> (w850:i32)
          n554 = Equal To 0?(x=w850) -> (x = 0?=w849:bool)
          n555 = case shown="真" w849 {
            frame False {
            }
            frame True {
              n556 = global read "全局 小时数据发送次数.vi" "小时数据发送次数"() -> (w852:i32)
              n557 = Increment(x=w852) -> (x+1=w851:i32)
              n558 = global write "全局 小时数据发送次数.vi" "小时数据发送次数"(w851) -> ()
            }
          }
        }
        frame "上传数据" {
          n559 = Index Array(array=w866, index #1=0 ("索引"), index #2=2 ("索引")) -> (element #1=w859:string)  [unwired: 1 out]
          n560 = call "规范时间戳.vi"("字符串"=w859) -> ("result string"=w857:string)  [unwired: 10 in]
          n561 = call "数据发送组合-20200825 (子VI).vi"("枚举"=T5."操作日志", "插值后的数组元素"=w854) -> ("字符串"=w853:string)  [unwired: 9 in]
          n562 = Format Into String(format string="DataTime=%s;", w857) -> (resulting string=w856:string)  [unwired: 2 in, 1 out]
          n563 = Concatenate Strings(w856, w853) -> (w861:string)
          n564 = Empty String/Path?(string/path=w861) -> (empty?=w865:bool)
          n565 = String Length(string=w861) -> (length=w863:i32)
          n566 = Decrement(x=w863) -> (x-1=w862:i32)
          n567 = String Subset(string=w861, length (rest)=w862) -> (substring=w860:string)  [unwired: 1 in]
          n568 = case shown="假" w865 {
            tunnel: [w871 ""] -> w864
            tunnel: w860 -> [w871 _]
            frame False {
              n569 = global read "全局 小时数据发送次数.vi" "小时数据发送次数"() -> (w870:i32)
              n570 = Increment(x=w870) -> (x+1=w869:i32)
              n571 = global write "全局 小时数据发送次数.vi" "小时数据发送次数"(w869) -> ()
            }
            frame True {
              n572 = global read "全局 小时数据发送次数.vi" "小时数据发送次数"() -> (w873:i32)
              n573 = Increment(x=w873) -> (x+1=w872:i32)
              n574 = global write "全局 小时数据发送次数.vi" "小时数据发送次数"(w872) -> ()
            }
          }
        }
        frame "返回执行结果" {
        }
      }
    }
    frame "3092日志信息" {
      n575 = global read "全局 小时数据发送次数.vi" "小时数据发送次数"() -> (w878:i32)
      n576 = global read "全局 所有参数.vi" "CODMn"() -> (w876:string[][])
      n577 = Index Array(array=w876, index (row)=w878) -> (element=w877:string[])  [unwired: 1 in]
      n578 = global read "全局1.vi" "枚举"() -> (w879:enum16{"返回请求应答", "上传数据", "返回执行结果"})
      n579 = case shown="\"上传数据\"" w879 {
        tunnel: ["QnRtn=1" w898 "ExeRtn=1"] -> w880
        tunnel: w877 -> [_ w900 _]
        frame "返回请求应答", Default {
          n580 = global read "全局 数据数组大小.vi" "数据数组大小"() -> (w883:i32)
          n581 = Equal To 0?(x=w883) -> (x = 0?=w882:bool)
          n582 = case shown="真" w882 {
            frame False {
            }
            frame True {
              n583 = global read "全局 小时数据发送次数.vi" "小时数据发送次数"() -> (w885:i32)
              n584 = Increment(x=w885) -> (x+1=w884:i32)
              n585 = global write "全局 小时数据发送次数.vi" "小时数据发送次数"(w884) -> ()
            }
          }
        }
        frame "上传数据" {
          n586 = Index Array(array=w900, index #1=0 ("索引")) -> (element #1=w893:string, element #2=w886:string, element #3=w888:string)  [unwired: 2 in]
          n587 = call "规范时间戳.vi"("字符串"=w893) -> ("result string"=w890:string)  [unwired: 10 in]
          n588 = Format Into String(format string="DataTime=%s;", w890) -> (resulting string=w891:string)  [unwired: 2 in, 1 out]
          n589 = Format Into String(format string="parameter=//%s//,content==//%s//;" ("格式字符串"), w886, w888) -> (resulting string=w887:string)  [unwired: 2 in, 1 out]
          n590 = Concatenate Strings(w891, w887) -> (w895:string)
          n591 = String Length(string=w895) -> (length=w897:i32)
          n592 = Empty String/Path?(string/path=w886) -> (empty?=w899:bool)
          n593 = Decrement(x=w897) -> (x-1=w896:i32)
          n594 = String Subset(string=w895, length (rest)=w896) -> (substring=w894:string)  [unwired: 1 in]
          n595 = case shown="假" w899 {
            tunnel: [w904 ""] -> w898
            tunnel: w894 -> [w904 _]
            frame False {
              n596 = global read "全局 小时数据发送次数.vi" "小时数据发送次数"() -> (w903:i32)
              n597 = Increment(x=w903) -> (x+1=w902:i32)
              n598 = global write "全局 小时数据发送次数.vi" "小时数据发送次数"(w902) -> ()
            }
            frame True {
              n599 = global read "全局 小时数据发送次数.vi" "小时数据发送次数"() -> (w906:i32)
              n600 = Increment(x=w906) -> (x+1=w905:i32)
              n601 = global write "全局 小时数据发送次数.vi" "小时数据发送次数"(w905) -> ()
            }
          }
        }
        frame "返回执行结果" {
        }
      }
    }
    frame "3093报警信息" {
      n602 = global read "全局 小时数据发送次数.vi" "小时数据发送次数"() -> (w911:i32)
      n603 = global read "全局 所有参数.vi" "CODMn"() -> (w909:string[][])
      n604 = Index Array(array=w909, index (row)=w911) -> (element=w910:string[])  [unwired: 1 in]
      n605 = global read "全局1.vi" "枚举"() -> (w912:enum16{"返回请求应答", "上传数据", "返回执行结果"})
      n606 = case shown="\"上传数据\"" w912 {
        tunnel: ["QnRtn=1" w933 "ExeRtn=1"] -> w913
        tunnel: w910 -> [_ w935 _]
        frame "返回请求应答", Default {
          n607 = global read "全局 数据数组大小.vi" "数据数组大小"() -> (w916:i32)
          n608 = Equal To 0?(x=w916) -> (x = 0?=w915:bool)
          n609 = case shown="真" w915 {
            frame False {
            }
            frame True {
              n610 = global read "全局 小时数据发送次数.vi" "小时数据发送次数"() -> (w918:i32)
              n611 = Increment(x=w918) -> (x+1=w917:i32)
              n612 = global write "全局 小时数据发送次数.vi" "小时数据发送次数"(w917) -> ()
            }
          }
        }
        frame "上传数据" {
          n613 = Index Array(array=w935, index #1=0 ("索引")) -> (element #1=w928:string, element #2=w922:string, element #3=w921:string, element #5=w920:string, element #6=w919:string)  [unwired: 5 in, 1 out]
          n614 = call "规范时间戳.vi"("字符串"=w928) -> ("result string"=w925:string)  [unwired: 10 in]
          n615 = Format Into String(format string="DataTime=%s;", w925) -> (resulting string=w926:string)  [unwired: 2 in, 1 out]
          n616 = Format Into String(format string="parameter=//%s//,code=//%s//,content=//%s//,state=%s;" ("格式字符串"), w922, w920, w921, w919) -> (resulting string=w923:string)  [unwired: 2 in, 1 out]
          n617 = Concatenate Strings(w926, w923) -> (w930:string)
          n618 = String Length(string=w930) -> (length=w932:i32)
          n619 = Empty String/Path?(string/path=w922) -> (empty?=w934:bool)
          n620 = Decrement(x=w932) -> (x-1=w931:i32)
          n621 = String Subset(string=w930, length (rest)=w931) -> (substring=w929:string)  [unwired: 1 in]
          n622 = case shown="假" w934 {
            tunnel: [w939 ""] -> w933
            tunnel: w929 -> [w939 _]
            frame False {
              n623 = global read "全局 小时数据发送次数.vi" "小时数据发送次数"() -> (w938:i32)
              n624 = Increment(x=w938) -> (x+1=w937:i32)
              n625 = global write "全局 小时数据发送次数.vi" "小时数据发送次数"(w937) -> ()
            }
            frame True {
              n626 = global read "全局 小时数据发送次数.vi" "小时数据发送次数"() -> (w941:i32)
              n627 = Increment(x=w941) -> (x+1=w940:i32)
              n628 = global write "全局 小时数据发送次数.vi" "小时数据发送次数"(w940) -> ()
            }
          }
        }
        frame "返回执行结果" {
        }
      }
    }
    frame "仪器参数" {
      n629 = case shown="\"氨氮\"" w947 {
        selector: w947 -> [w951 _ _ _ _ _ _ _ _ _ _ _ _ _ _ _ _ _ _ _ _ _ _ _ _ _ _ _ _ _ _ _]
        tunnel: [w951 w954 w958 w962 w966 w970 w974 w978 w982 w986 w990 w994 w998 w1002 w1006 w1010 w1014 w1018 w1022 w1026 w1030 w1034 w1038 w1042 w1046 w1050 w1054 w1058 w1062 w1066 w1070 w1074] -> w946
        tunnel: [1.0 ("风向") w952 w956 w960 w964 w968 w972 w976 w980 w984 w988 w992 w996 w1000 w1004 w1008 w1012 w1016 w1020 w1024 w1028 w1032 w1036 w1040 w1044 w1048 w1052 w1056 w1060 w1064 w1068 w1072] -> _
        frame "假", Default {
        }
        frame "CODMn" {
          n630 = global read "断电保存全局.vi" "因子编码簇"() -> (w955:T7)
          n631 = global read "断电保存全局.vi" "参数系数簇"() -> (w953:T8)
          n632 = Unbundle By Name(w955) -> ("CODMn"=w954:string)
          n633 = Unbundle By Name(w953) -> ("CODMn"=w952:dbl)
        }
        frame "CODCr" {
          n634 = global read "断电保存全局.vi" "参数系数簇"() -> (w957:T8)
          n635 = global read "断电保存全局.vi" "因子编码簇"() -> (w959:T7)
          n636 = Unbundle By Name(w957) -> ("CODCr"=w956:dbl)
          n637 = Unbundle By Name(w959) -> ("CODCr"=w958:string)
        }
        frame "DO" {
          n638 = global read "断电保存全局.vi" "参数系数簇"() -> (w961:T8)
          n639 = global read "断电保存全局.vi" "因子编码簇"() -> (w963:T7)
          n640 = Unbundle By Name(w961) -> ("DO"=w960:dbl)
          n641 = Unbundle By Name(w963) -> ("DO"=w962:string)
        }
        frame "铜" {
          n642 = global read "断电保存全局.vi" "参数系数簇"() -> (w965:T8)
          n643 = global read "断电保存全局.vi" "因子编码簇"() -> (w967:T7)
          n644 = Unbundle By Name(w965) -> ("铜"=w964:dbl)
          n645 = Unbundle By Name(w967) -> ("铜"=w966:string)
        }
        frame "PH" {
          n646 = global read "断电保存全局.vi" "参数系数簇"() -> (w969:T8)
          n647 = global read "断电保存全局.vi" "因子编码簇"() -> (w971:T7)
          n648 = Unbundle By Name(w969) -> ("PH"=w968:dbl)
          n649 = Unbundle By Name(w971) -> ("PH"=w970:string)
        }
        frame "氨氮" {
          n650 = global read "断电保存全局.vi" "参数系数簇"() -> (w973:T8)
          n651 = global read "断电保存全局.vi" "因子编码簇"() -> (w975:T7)
          n652 = Unbundle By Name(w973) -> ("氨氮"=w972:dbl)
          n653 = Unbundle By Name(w975) -> ("氨氮"=w974:string)
        }
        frame "比电导率" {
          n654 = global read "断电保存全局.vi" "参数系数簇"() -> (w977:T8)
          n655 = global read "断电保存全局.vi" "因子编码簇"() -> (w979:T7)
          n656 = Unbundle By Name(w977) -> ("比电导率"=w976:dbl)
          n657 = Unbundle By Name(w979) -> ("比电导率"=w978:string)
        }
        frame "水温" {
          n658 = global read "断电保存全局.vi" "参数系数簇"() -> (w981:T8)
          n659 = global read "断电保存全局.vi" "因子编码簇"() -> (w983:T7)
          n660 = Unbundle By Name(w981) -> ("水温"=w980:dbl)
          n661 = Unbundle By Name(w983) -> ("水温"=w982:string)
        }
        frame "COD" {
          n662 = global read "断电保存全局.vi" "参数系数簇"() -> (w985:T8)
          n663 = global read "断电保存全局.vi" "因子编码簇"() -> (w987:T7)
          n664 = Unbundle By Name(w985) -> ("COD"=w984:dbl)
          n665 = Unbundle By Name(w987) -> ("COD"=w986:string)
        }
        frame "浊度" {
          n666 = global read "断电保存全局.vi" "参数系数簇"() -> (w989:T8)
          n667 = global read "断电保存全局.vi" "因子编码簇"() -> (w991:T7)
          n668 = Unbundle By Name(w989) -> ("浊度"=w988:dbl)
          n669 = Unbundle By Name(w991) -> ("浊度"=w990:string)
        }
        frame "总氮" {
          n670 = global read "断电保存全局.vi" "参数系数簇"() -> (w993:T8)
          n671 = global read "断电保存全局.vi" "因子编码簇"() -> (w995:T7)
          n672 = Unbundle By Name(w993) -> ("总氮"=w992:dbl)
          n673 = Unbundle By Name(w995) -> ("总氮"=w994:string)
        }
        frame "总磷" {
          n674 = global read "断电保存全局.vi" "参数系数簇"() -> (w997:T8)
          n675 = global read "断电保存全局.vi" "因子编码簇"() -> (w999:T7)
          n676 = Unbundle By Name(w997) -> ("总磷"=w996:dbl)
          n677 = Unbundle By Name(w999) -> ("总磷"=w998:string)
        }
        frame "叶绿素a" {
          n678 = global read "断电保存全局.vi" "参数系数簇"() -> (w1001:T8)
          n679 = global read "断电保存全局.vi" "因子编码簇"() -> (w1003:T7)
          n680 = Unbundle By Name(w1001) -> ("叶绿素a"=w1000:dbl)
          n681 = Unbundle By Name(w1003) -> ("叶绿素a"=w1002:string)
        }
        frame "藻密度" {
          n682 = global read "断电保存全局.vi" "参数系数簇"() -> (w1005:T8)
          n683 = global read "断电保存全局.vi" "因子编码簇"() -> (w1007:T7)
          n684 = Unbundle By Name(w1005) -> ("藻密度"=w1004:dbl)
          n685 = Unbundle By Name(w1007) -> ("藻密度"=w1006:string)
        }
        frame "水位" {
          n686 = global read "断电保存全局.vi" "因子编码簇"() -> (w1011:T7)
          n687 = global read "断电保存全局.vi" "参数系数簇"() -> (w1009:T8)
          n688 = Unbundle By Name(w1011) -> ("水位"=w1010:string)
          n689 = Unbundle By Name(w1009) -> ("水位"=w1008:dbl)
        }
        frame "流速" {
          n690 = global read "断电保存全局.vi" "参数系数簇"() -> (w1013:T8)
          n691 = global read "断电保存全局.vi" "因子编码簇"() -> (w1015:T7)
          n692 = Unbundle By Name(w1013) -> ("流速"=w1012:dbl)
          n693 = Unbundle By Name(w1015) -> ("流速"=w1014:string)
        }
        frame "瞬时流量" {
          n694 = global read "断电保存全局.vi" "参数系数簇"() -> (w1017:T8)
          n695 = global read "断电保存全局.vi" "因子编码簇"() -> (w1019:T7)
          n696 = Unbundle By Name(w1017) -> ("瞬时流量"=w1016:dbl)
          n697 = Unbundle By Name(w1019) -> ("瞬时流量"=w1018:string)
        }
        frame "累积流量" {
          n698 = global read "断电保存全局.vi" "参数系数簇"() -> (w1021:T8)
          n699 = global read "断电保存全局.vi" "因子编码簇"() -> (w1023:T7)
          n700 = Unbundle By Name(w1021) -> ("累积流量"=w1020:dbl)
          n701 = Unbundle By Name(w1023) -> ("累积流量"=w1022:string)
        }
        frame "亚硝酸盐" {
          n702 = global read "断电保存全局.vi" "参数系数簇"() -> (w1025:T8)
          n703 = global read "断电保存全局.vi" "因子编码簇"() -> (w1027:T7)
          n704 = Unbundle By Name(w1025) -> ("亚硝酸盐"=w1024:dbl)
          n705 = Unbundle By Name(w1027) -> ("亚硝酸盐"=w1026:string)
        }
        frame "硫化物" {
          n706 = global read "断电保存全局.vi" "参数系数簇"() -> (w1029:T8)
          n707 = global read "断电保存全局.vi" "因子编码簇"() -> (w1031:T7)
          n708 = Unbundle By Name(w1029) -> ("硫化物"=w1028:dbl)
          n709 = Unbundle By Name(w1031) -> ("硫化物"=w1030:string)
        }
        frame "ORP" {
          n710 = global read "断电保存全局.vi" "参数系数簇"() -> (w1033:T8)
          n711 = global read "断电保存全局.vi" "因子编码簇"() -> (w1035:T7)
          n712 = Unbundle By Name(w1033) -> ("ORP"=w1032:dbl)
          n713 = Unbundle By Name(w1035) -> ("ORP"=w1034:string)
        }
        frame "铅" {
          n714 = global read "断电保存全局.vi" "参数系数簇"() -> (w1037:T8)
          n715 = global read "断电保存全局.vi" "因子编码簇"() -> (w1039:T7)
          n716 = Unbundle By Name(w1039) -> ("铅"=w1038:string)
          n717 = Unbundle By Name(w1037) -> ("铅"=w1036:dbl)
        }
        frame "镉" {
          n718 = global read "断电保存全局.vi" "参数系数簇"() -> (w1041:T8)
          n719 = global read "断电保存全局.vi" "因子编码簇"() -> (w1043:T7)
          n720 = Unbundle By Name(w1041) -> ("镉"=w1040:dbl)
          n721 = Unbundle By Name(w1043) -> ("镉"=w1042:string)
        }
        frame "锌" {
          n722 = global read "断电保存全局.vi" "参数系数簇"() -> (w1045:T8)
          n723 = global read "断电保存全局.vi" "因子编码簇"() -> (w1047:T7)
          n724 = Unbundle By Name(w1045) -> ("锌"=w1044:dbl)
          n725 = Unbundle By Name(w1047) -> ("锌"=w1046:string)
        }
        frame "镍" {
          n726 = global read "断电保存全局.vi" "参数系数簇"() -> (w1049:T8)
          n727 = global read "断电保存全局.vi" "因子编码簇"() -> (w1051:T7)
          n728 = Unbundle By Name(w1049) -> ("镍"=w1048:dbl)
          n729 = Unbundle By Name(w1051) -> ("镍"=w1050:string)
        }
        frame "锰" {
          n730 = global read "断电保存全局.vi" "参数系数簇"() -> (w1053:T8)
          n731 = global read "断电保存全局.vi" "因子编码簇"() -> (w1055:T7)
          n732 = Unbundle By Name(w1055) -> ("锰"=w1054:string)
          n733 = Unbundle By Name(w1053) -> ("锰"=w1052:dbl)
        }
        frame "汞" {
          n734 = global read "断电保存全局.vi" "参数系数簇"() -> (w1057:T8)
          n735 = global read "断电保存全局.vi" "因子编码簇"() -> (w1059:T7)
          n736 = Unbundle By Name(w1059) -> ("汞"=w1058:string)
          n737 = Unbundle By Name(w1057) -> ("汞"=w1056:dbl)
        }
        frame "气温" {
          n738 = global read "断电保存全局.vi" "因子编码簇"() -> (w1063:T7)
          n739 = global read "断电保存全局.vi" "参数系数簇"() -> (w1061:T8)
          n740 = Unbundle By Name(w1063) -> ("气温"=w1062:string)
          n741 = Unbundle By Name(w1061) -> ("气温"=w1060:dbl)
        }
        frame "气压" {
          n742 = global read "断电保存全局.vi" "参数系数簇"() -> (w1065:T8)
          n743 = global read "断电保存全局.vi" "因子编码簇"() -> (w1067:T7)
          n744 = Unbundle By Name(w1065) -> ("气压"=w1064:dbl)
          n745 = Unbundle By Name(w1067) -> ("气压"=w1066:string)
        }
        frame "风速" {
          n746 = global read "断电保存全局.vi" "参数系数簇"() -> (w1069:T8)
          n747 = global read "断电保存全局.vi" "因子编码簇"() -> (w1071:T7)
          n748 = Unbundle By Name(w1069) -> ("风速"=w1068:dbl)
          n749 = Unbundle By Name(w1071) -> ("风速"=w1070:string)
        }
        frame "风向" {
          n750 = global read "断电保存全局.vi" "参数系数簇"() -> (w1073:T8)
          n751 = global read "断电保存全局.vi" "因子编码簇"() -> (w1075:T7)
          n752 = Unbundle By Name(w1075) -> ("风向"=w1074:string)
          n753 = Unbundle By Name(w1073) -> ("风向"=w1072:dbl)
        }
      }
      n754 = global read "全局1.vi" "枚举"() -> (w948:enum16{"返回请求应答", "上传数据", "返回执行结果"})
      n755 = case shown="\"上传数据\"" w948 {
        tunnel: ["QnRtn=1" w1093 "ExeRtn=1"] -> w949
        tunnel: w945 -> [_ w1085 _]
        tunnel: w946 -> [_ w1084 _]
        tunnel: w944 -> [_ w1082 _]
        frame "返回请求应答", Default {
          n756 = global read "全局 数据数组大小.vi" "数据数组大小"() -> (w1078:i32)
          n757 = Equal To 0?(x=w1078) -> (x = 0?=w1077:bool)
          n758 = case shown="真" w1077 {
            frame False {
            }
            frame True {
              n759 = global read "全局 小时数据发送次数.vi" "小时数据发送次数"() -> (w1080:i32)
              n760 = Increment(x=w1080) -> (x+1=w1079:i32)
              n761 = global write "全局 小时数据发送次数.vi" "小时数据发送次数"(w1079) -> ()
            }
          }
        }
        frame "上传数据" {
          n762 = Index Array(array=w1085) -> (element=w1086:string)  [unwired: 1 in]
          n763 = case shown="\"原始时间\"" w1082 {
            tunnel: [w1096 w1098] -> w1087
            tunnel: w1086 -> [w1095 w1097]
            frame "精确到小时", Default {
              n764 = call "规范小时时间戳.vi"("字符串"=w1095) -> ("result string"=w1096:string)  [unwired: 10 in]
            }
            frame "原始时间" {
              n765 = call "日期字符串格式至时间格式转换(子VI).vi"("data[0]"=w1097) -> ("time stamp"=w1100:timestamp)  [unwired: 10 in]
              n766 = Seconds To Date/Time(time stamp (now)=w1100) -> (date time rec=w1099:T9)  [unwired: 1 in]
              n767 = Date/Time To Seconds(2:w1099) -> (0:w1101:timestamp)  [unwired: 1 in]
              n768 = Format Date/Time String(time format string (%c)="%Y%m%d%H%M%S" ("时间格式字符串(%c)"), seconds (now)=w1101) -> (date/time string=w1098:string)  [unwired: 1 in]
            }
          }
          n769 = call "关键参数组合 (子VI).vi"("table"="仪器参数", "因子编码"=w1084, "data"=w1085) -> ("字符串"=w1081:string)  [unwired: 8 in]
          n770 = Format Into String(format string="DataTime=%s;%s" ("格式字符串"), w1087, w1081) -> (resulting string=w1089:string)  [unwired: 2 in, 1 out]
          n771 = String Length(string=w1089) -> (length=w1090:i32)
          n772 = Decrement(x=w1090) -> (x-1=w1091:i32)
          n773 = String Subset(string=w1089, length (rest)=w1091) -> (substring=w1088:string)  [unwired: 1 in]
          n774 = Empty String/Path?(string/path=w1081) -> (empty?=w1094:bool)
          n775 = case shown="假" w1094 {
            tunnel: [w1103 ""] -> w1093
            tunnel: w1088 -> [w1103 _]
            frame False {
            }
            frame True {
            }
          }
        }
        frame "返回执行结果" {
        }
      }
    }
    frame "采配水仪器参数" {
      n776 = global read "全局1.vi" "枚举"() -> (w1109:enum16{"返回请求应答", "上传数据", "返回执行结果"})
      n777 = case shown="\"上传数据\"" w1109 {
        tunnel: ["QnRtn=1" w1134 "ExeRtn=1"] -> w1110
        tunnel: w1108 -> [_ w1122 _]
        tunnel: "w00000" -> [_ w1123 _]
        tunnel: w1107 -> [_ w1126 _]
        frame "返回请求应答", Default {
          n778 = global read "全局 数据数组大小.vi" "数据数组大小"() -> (w1113:i32)
          n779 = Equal To 0?(x=w1113) -> (x = 0?=w1112:bool)
          n780 = case shown="真" w1112 {
            frame False {
            }
            frame True {
              n781 = global read "全局 小时数据发送次数.vi" "小时数据发送次数"() -> (w1115:i32)
              n782 = Increment(x=w1115) -> (x+1=w1114:i32)
              n783 = global write "全局 小时数据发送次数.vi" "小时数据发送次数"(w1114) -> ()
            }
          }
        }
        frame "上传数据" {
          n784 = Index Array(array=w1122, index #1=2 ("索引"), index #2=3 ("索引"), index #3=4 ("索引")) -> (element #1=w1118:string, element #2=w1117:string, element #3=w1116:string)
          n785 = Index Array(array=w1122) -> (element=w1127:string)  [unwired: 1 in]
          n786 = case shown="\"原始时间\"" w1126 {
            tunnel: [w1137 w1139] -> w1128
            tunnel: w1127 -> [w1136 w1138]
            frame "精确到小时", Default {
              n787 = call "规范小时时间戳.vi"("字符串"=w1136) -> ("result string"=w1137:string)  [unwired: 10 in]
            }
            frame "原始时间" {
              n788 = call "日期字符串格式至时间格式转换(子VI).vi"("data[0]"=w1138) -> ("time stamp"=w1141:timestamp)  [unwired: 10 in]
              n789 = Seconds To Date/Time(time stamp (now)=w1141) -> (date time rec=w1140:T9)  [unwired: 1 in]
              n790 = Date/Time To Seconds(2:w1140) -> (0:w1142:timestamp)  [unwired: 1 in]
              n791 = Format Date/Time String(time format string (%c)="%Y%m%d%H%M%S" ("时间格式字符串(%c)"), seconds (now)=w1142) -> (date/time string=w1139:string)  [unwired: 1 in]
            }
          }
          n792 = Format Into String(format string="PolId=%s,i13111-Info=%s,i13112-Info=%s,i13113-Info=%s;", w1123, w1118, w1117, w1116) -> (resulting string=w1124:string)  [unwired: 2 in, 1 out]
          n793 = Format Into String(format string="DataTime=%s;%s" ("格式字符串"), w1128, w1124) -> (resulting string=w1130:string)  [unwired: 2 in, 1 out]
          n794 = String Length(string=w1130) -> (length=w1131:i32)
          n795 = Decrement(x=w1131) -> (x-1=w1132:i32)
          n796 = String Subset(string=w1130, length (rest)=w1132) -> (substring=w1129:string)  [unwired: 1 in]
          n797 = Empty String/Path?(string/path=w1124) -> (empty?=w1135:bool)
          n798 = case shown="假" w1135 {
            tunnel: [w1144 ""] -> w1134
            tunnel: w1129 -> [w1144 _]
            frame False {
            }
            frame True {
            }
          }
        }
        frame "返回执行结果" {
        }
      }
    }
    frame "3091校准信息" {
      n799 = case shown="\"CODMn\"" w1150 {
        selector: w1150 -> [w1154 _ _ _ _ _ _ _ _ _ _ _ _ _ _ _ _ _ _ _ _ _ _ _ _ _ _ _ _ _ _ _]
        tunnel: [w1154 w1157 w1161 w1165 w1169 w1173 w1177 w1181 w1185 w1189 w1193 w1197 w1201 w1205 w1209 w1213 w1217 w1221 w1225 w1229 w1233 w1237 w1241 w1245 w1249 w1253 w1257 w1261 w1265 w1269 w1273 w1277] -> w1149
        tunnel: [1.0 ("风向") w1155 w1159 w1163 w1167 w1171 w1175 w1179 w1183 w1187 w1191 w1195 w1199 w1203 w1207 w1211 w1215 w1219 w1223 w1227 w1231 w1235 w1239 w1243 w1247 w1251 w1255 w1259 w1263 w1267 w1271 w1275] -> _
        frame "假", Default {
        }
        frame "CODMn" {
          n800 = global read "断电保存全局.vi" "因子编码簇"() -> (w1158:T7)
          n801 = global read "断电保存全局.vi" "参数系数簇"() -> (w1156:T8)
          n802 = Unbundle By Name(w1158) -> ("CODMn"=w1157:string)
          n803 = Unbundle By Name(w1156) -> ("CODMn"=w1155:dbl)
        }
        frame "CODCr" {
          n804 = global read "断电保存全局.vi" "参数系数簇"() -> (w1160:T8)
          n805 = global read "断电保存全局.vi" "因子编码簇"() -> (w1162:T7)
          n806 = Unbundle By Name(w1160) -> ("CODCr"=w1159:dbl)
          n807 = Unbundle By Name(w1162) -> ("CODCr"=w1161:string)
        }
        frame "DO" {
          n808 = global read "断电保存全局.vi" "参数系数簇"() -> (w1164:T8)
          n809 = global read "断电保存全局.vi" "因子编码簇"() -> (w1166:T7)
          n810 = Unbundle By Name(w1164) -> ("DO"=w1163:dbl)
          n811 = Unbundle By Name(w1166) -> ("DO"=w1165:string)
        }
        frame "铜" {
          n812 = global read "断电保存全局.vi" "参数系数簇"() -> (w1168:T8)
          n813 = global read "断电保存全局.vi" "因子编码簇"() -> (w1170:T7)
          n814 = Unbundle By Name(w1168) -> ("铜"=w1167:dbl)
          n815 = Unbundle By Name(w1170) -> ("铜"=w1169:string)
        }
        frame "PH" {
          n816 = global read "断电保存全局.vi" "参数系数簇"() -> (w1172:T8)
          n817 = global read "断电保存全局.vi" "因子编码簇"() -> (w1174:T7)
          n818 = Unbundle By Name(w1172) -> ("PH"=w1171:dbl)
          n819 = Unbundle By Name(w1174) -> ("PH"=w1173:string)
        }
        frame "氨氮" {
          n820 = global read "断电保存全局.vi" "参数系数簇"() -> (w1176:T8)
          n821 = global read "断电保存全局.vi" "因子编码簇"() -> (w1178:T7)
          n822 = Unbundle By Name(w1176) -> ("氨氮"=w1175:dbl)
          n823 = Unbundle By Name(w1178) -> ("氨氮"=w1177:string)
        }
        frame "比电导率" {
          n824 = global read "断电保存全局.vi" "参数系数簇"() -> (w1180:T8)
          n825 = global read "断电保存全局.vi" "因子编码簇"() -> (w1182:T7)
          n826 = Unbundle By Name(w1180) -> ("比电导率"=w1179:dbl)
          n827 = Unbundle By Name(w1182) -> ("比电导率"=w1181:string)
        }
        frame "水温" {
          n828 = global read "断电保存全局.vi" "参数系数簇"() -> (w1184:T8)
          n829 = global read "断电保存全局.vi" "因子编码簇"() -> (w1186:T7)
          n830 = Unbundle By Name(w1184) -> ("水温"=w1183:dbl)
          n831 = Unbundle By Name(w1186) -> ("水温"=w1185:string)
        }
        frame "COD" {
          n832 = global read "断电保存全局.vi" "参数系数簇"() -> (w1188:T8)
          n833 = global read "断电保存全局.vi" "因子编码簇"() -> (w1190:T7)
          n834 = Unbundle By Name(w1188) -> ("COD"=w1187:dbl)
          n835 = Unbundle By Name(w1190) -> ("COD"=w1189:string)
        }
        frame "浊度" {
          n836 = global read "断电保存全局.vi" "参数系数簇"() -> (w1192:T8)
          n837 = global read "断电保存全局.vi" "因子编码簇"() -> (w1194:T7)
          n838 = Unbundle By Name(w1192) -> ("浊度"=w1191:dbl)
          n839 = Unbundle By Name(w1194) -> ("浊度"=w1193:string)
        }
        frame "总氮" {
          n840 = global read "断电保存全局.vi" "参数系数簇"() -> (w1196:T8)
          n841 = global read "断电保存全局.vi" "因子编码簇"() -> (w1198:T7)
          n842 = Unbundle By Name(w1196) -> ("总氮"=w1195:dbl)
          n843 = Unbundle By Name(w1198) -> ("总氮"=w1197:string)
        }
        frame "总磷" {
          n844 = global read "断电保存全局.vi" "参数系数簇"() -> (w1200:T8)
          n845 = global read "断电保存全局.vi" "因子编码簇"() -> (w1202:T7)
          n846 = Unbundle By Name(w1200) -> ("总磷"=w1199:dbl)
          n847 = Unbundle By Name(w1202) -> ("总磷"=w1201:string)
        }
        frame "叶绿素a" {
          n848 = global read "断电保存全局.vi" "参数系数簇"() -> (w1204:T8)
          n849 = global read "断电保存全局.vi" "因子编码簇"() -> (w1206:T7)
          n850 = Unbundle By Name(w1204) -> ("叶绿素a"=w1203:dbl)
          n851 = Unbundle By Name(w1206) -> ("叶绿素a"=w1205:string)
        }
        frame "藻密度" {
          n852 = global read "断电保存全局.vi" "参数系数簇"() -> (w1208:T8)
          n853 = global read "断电保存全局.vi" "因子编码簇"() -> (w1210:T7)
          n854 = Unbundle By Name(w1208) -> ("藻密度"=w1207:dbl)
          n855 = Unbundle By Name(w1210) -> ("藻密度"=w1209:string)
        }
        frame "水位" {
          n856 = global read "断电保存全局.vi" "因子编码簇"() -> (w1214:T7)
          n857 = global read "断电保存全局.vi" "参数系数簇"() -> (w1212:T8)
          n858 = Unbundle By Name(w1214) -> ("水位"=w1213:string)
          n859 = Unbundle By Name(w1212) -> ("水位"=w1211:dbl)
        }
        frame "流速" {
          n860 = global read "断电保存全局.vi" "参数系数簇"() -> (w1216:T8)
          n861 = global read "断电保存全局.vi" "因子编码簇"() -> (w1218:T7)
          n862 = Unbundle By Name(w1216) -> ("流速"=w1215:dbl)
          n863 = Unbundle By Name(w1218) -> ("流速"=w1217:string)
        }
        frame "瞬时流量" {
          n864 = global read "断电保存全局.vi" "参数系数簇"() -> (w1220:T8)
          n865 = global read "断电保存全局.vi" "因子编码簇"() -> (w1222:T7)
          n866 = Unbundle By Name(w1220) -> ("瞬时流量"=w1219:dbl)
          n867 = Unbundle By Name(w1222) -> ("瞬时流量"=w1221:string)
        }
        frame "累积流量" {
          n868 = global read "断电保存全局.vi" "参数系数簇"() -> (w1224:T8)
          n869 = global read "断电保存全局.vi" "因子编码簇"() -> (w1226:T7)
          n870 = Unbundle By Name(w1224) -> ("累积流量"=w1223:dbl)
          n871 = Unbundle By Name(w1226) -> ("累积流量"=w1225:string)
        }
        frame "亚硝酸盐" {
          n872 = global read "断电保存全局.vi" "参数系数簇"() -> (w1228:T8)
          n873 = global read "断电保存全局.vi" "因子编码簇"() -> (w1230:T7)
          n874 = Unbundle By Name(w1228) -> ("亚硝酸盐"=w1227:dbl)
          n875 = Unbundle By Name(w1230) -> ("亚硝酸盐"=w1229:string)
        }
        frame "硫化物" {
          n876 = global read "断电保存全局.vi" "参数系数簇"() -> (w1232:T8)
          n877 = global read "断电保存全局.vi" "因子编码簇"() -> (w1234:T7)
          n878 = Unbundle By Name(w1232) -> ("硫化物"=w1231:dbl)
          n879 = Unbundle By Name(w1234) -> ("硫化物"=w1233:string)
        }
        frame "ORP" {
          n880 = global read "断电保存全局.vi" "参数系数簇"() -> (w1236:T8)
          n881 = global read "断电保存全局.vi" "因子编码簇"() -> (w1238:T7)
          n882 = Unbundle By Name(w1236) -> ("ORP"=w1235:dbl)
          n883 = Unbundle By Name(w1238) -> ("ORP"=w1237:string)
        }
        frame "铅" {
          n884 = global read "断电保存全局.vi" "参数系数簇"() -> (w1240:T8)
          n885 = global read "断电保存全局.vi" "因子编码簇"() -> (w1242:T7)
          n886 = Unbundle By Name(w1242) -> ("铅"=w1241:string)
          n887 = Unbundle By Name(w1240) -> ("铅"=w1239:dbl)
        }
        frame "镉" {
          n888 = global read "断电保存全局.vi" "参数系数簇"() -> (w1244:T8)
          n889 = global read "断电保存全局.vi" "因子编码簇"() -> (w1246:T7)
          n890 = Unbundle By Name(w1244) -> ("镉"=w1243:dbl)
          n891 = Unbundle By Name(w1246) -> ("镉"=w1245:string)
        }
        frame "锌" {
          n892 = global read "断电保存全局.vi" "参数系数簇"() -> (w1248:T8)
          n893 = global read "断电保存全局.vi" "因子编码簇"() -> (w1250:T7)
          n894 = Unbundle By Name(w1248) -> ("锌"=w1247:dbl)
          n895 = Unbundle By Name(w1250) -> ("锌"=w1249:string)
        }
        frame "镍" {
          n896 = global read "断电保存全局.vi" "参数系数簇"() -> (w1252:T8)
          n897 = global read "断电保存全局.vi" "因子编码簇"() -> (w1254:T7)
          n898 = Unbundle By Name(w1252) -> ("镍"=w1251:dbl)
          n899 = Unbundle By Name(w1254) -> ("镍"=w1253:string)
        }
        frame "锰" {
          n900 = global read "断电保存全局.vi" "参数系数簇"() -> (w1256:T8)
          n901 = global read "断电保存全局.vi" "因子编码簇"() -> (w1258:T7)
          n902 = Unbundle By Name(w1258) -> ("锰"=w1257:string)
          n903 = Unbundle By Name(w1256) -> ("锰"=w1255:dbl)
        }
        frame "汞" {
          n904 = global read "断电保存全局.vi" "参数系数簇"() -> (w1260:T8)
          n905 = global read "断电保存全局.vi" "因子编码簇"() -> (w1262:T7)
          n906 = Unbundle By Name(w1262) -> ("汞"=w1261:string)
          n907 = Unbundle By Name(w1260) -> ("汞"=w1259:dbl)
        }
        frame "气温" {
          n908 = global read "断电保存全局.vi" "因子编码簇"() -> (w1266:T7)
          n909 = global read "断电保存全局.vi" "参数系数簇"() -> (w1264:T8)
          n910 = Unbundle By Name(w1266) -> ("气温"=w1265:string)
          n911 = Unbundle By Name(w1264) -> ("气温"=w1263:dbl)
        }
        frame "气压" {
          n912 = global read "断电保存全局.vi" "参数系数簇"() -> (w1268:T8)
          n913 = global read "断电保存全局.vi" "因子编码簇"() -> (w1270:T7)
          n914 = Unbundle By Name(w1268) -> ("气压"=w1267:dbl)
          n915 = Unbundle By Name(w1270) -> ("气压"=w1269:string)
        }
        frame "风速" {
          n916 = global read "断电保存全局.vi" "参数系数簇"() -> (w1272:T8)
          n917 = global read "断电保存全局.vi" "因子编码簇"() -> (w1274:T7)
          n918 = Unbundle By Name(w1272) -> ("风速"=w1271:dbl)
          n919 = Unbundle By Name(w1274) -> ("风速"=w1273:string)
        }
        frame "风向" {
          n920 = global read "断电保存全局.vi" "参数系数簇"() -> (w1276:T8)
          n921 = global read "断电保存全局.vi" "因子编码簇"() -> (w1278:T7)
          n922 = Unbundle By Name(w1278) -> ("风向"=w1277:string)
          n923 = Unbundle By Name(w1276) -> ("风向"=w1275:dbl)
        }
      }
      n924 = global read "全局1.vi" "枚举"() -> (w1151:enum16{"返回请求应答", "上传数据", "返回执行结果"})
      n925 = case shown="\"上传数据\"" w1151 {
        tunnel: ["QnRtn=1" w1295 "ExeRtn=1"] -> w1152
        tunnel: w1148 -> [_ w1285 _]
        tunnel: w1149 -> [_ w1284 _]
        tunnel: w1147 -> [_ w1287 _]
        frame "返回请求应答", Default {
          n926 = global read "全局 数据数组大小.vi" "数据数组大小"() -> (w1281:i32)
          n927 = Equal To 0?(x=w1281) -> (x = 0?=w1280:bool)
          n928 = case shown="真" w1280 {
            frame False {
            }
            frame True {
              n929 = global read "全局 小时数据发送次数.vi" "小时数据发送次数"() -> (w1283:i32)
              n930 = Increment(x=w1283) -> (x+1=w1282:i32)
              n931 = global write "全局 小时数据发送次数.vi" "小时数据发送次数"(w1282) -> ()
            }
          }
        }
        frame "上传数据" {
          n932 = Index Array(array=w1285) -> (element=w1288:string)  [unwired: 1 in]
          n933 = case shown="\"原始时间\"" w1287 {
            tunnel: [w1298 w1300] -> w1289
            tunnel: w1288 -> [w1297 w1299]
            frame "精确到小时", Default {
              n934 = call "规范小时时间戳.vi"("字符串"=w1297) -> ("result string"=w1298:string)  [unwired: 10 in]
            }
            frame "原始时间" {
              n935 = call "日期字符串格式至时间格式转换(子VI).vi"("data[0]"=w1299) -> ("time stamp"=w1302:timestamp)  [unwired: 10 in]
              n936 = Seconds To Date/Time(time stamp (now)=w1302) -> (date time rec=w1301:T9)  [unwired: 1 in]
              n937 = Date/Time To Seconds(2:w1301) -> (0:w1303:timestamp)  [unwired: 1 in]
              n938 = Format Date/Time String(time format string (%c)="%Y%m%d%H%M%S" ("时间格式字符串(%c)"), seconds (now)=w1303) -> (date/time string=w1300:string)  [unwired: 1 in]
            }
          }
          n939 = call "校准信息组合 (子VI).vi"("因子编码"=w1284, "data"=w1285) -> ("字符串"=w1286:string)  [unwired: 9 in]
          n940 = Format Into String(format string="DataTime=%s;%s" ("格式字符串"), w1289, w1286) -> (resulting string=w1291:string)  [unwired: 2 in, 1 out]
          n941 = String Length(string=w1291) -> (length=w1292:i32)
          n942 = Decrement(x=w1292) -> (x-1=w1293:i32)
          n943 = String Subset(string=w1291, length (rest)=w1293) -> (substring=w1290:string)  [unwired: 1 in]
          n944 = Empty String/Path?(string/path=w1286) -> (empty?=w1296:bool)
          n945 = case shown="假" w1296 {
            tunnel: [w1305 ""] -> w1295
            tunnel: w1290 -> [w1305 _]
            frame False {
            }
            frame True {
            }
          }
        }
        frame "返回执行结果" {
        }
      }
    }
    frame "3090仪器参数" {
      n946 = global read "全局 小时数据发送次数.vi" "小时数据发送次数"() -> (w1310:i32)
      n947 = Index Array(array=w1312, index (row)=w1310) -> (element=w1309:string[])  [unwired: 1 in]
      n948 = global read "全局1.vi" "枚举"() -> (w1311:enum16{"返回请求应答", "上传数据", "返回执行结果"})
      n949 = case shown="\"上传数据\"" w1311 {
        tunnel: ["QnRtn=1" w1330 "ExeRtn=1"] -> w1313
        tunnel: w1309 -> [_ w1327 _]
        tunnel: w1308 -> [_ w1320 _]
        frame "返回请求应答", Default {
          n950 = global read "全局 数据数组大小.vi" "数据数组大小"() -> (w1316:i32)
          n951 = Equal To 0?(x=w1316) -> (x = 0?=w1315:bool)
          n952 = case shown="真" w1315 {
            frame False {
            }
            frame True {
              n953 = global read "全局 小时数据发送次数.vi" "小时数据发送次数"() -> (w1318:i32)
              n954 = Increment(x=w1318) -> (x+1=w1317:i32)
              n955 = global write "全局 小时数据发送次数.vi" "小时数据发送次数"(w1317) -> ()
            }
          }
        }
        frame "上传数据" {
          n956 = Index Array(array=w1327) -> (element=w1326:string)  [unwired: 1 in]
          n957 = call "规范时间戳.vi"("字符串"=w1326) -> ("result string"=w1328:string)  [unwired: 10 in]
          n958 = call "数据发送组合-20200825 (子VI).vi"("枚举"=T6."3090仪器参数", "插值后的数组元素"=w1320) -> ("字符串"=w1319:string)  [unwired: 9 in]
          n959 = Format Into String(format string="DataTime=%s;%s" ("格式字符串"), w1328, w1319) -> (resulting string=w1323:string)  [unwired: 2 in, 1 out]
          n960 = String Length(string=w1323) -> (length=w1324:i32)
          n961 = Decrement(x=w1324) -> (x-1=w1325:i32)
          n962 = String Subset(string=w1323, length (rest)=w1325) -> (substring=w1322:string)  [unwired: 1 in]
          n963 = Empty String/Path?(string/path=w1322) -> (empty?=w1331:bool)
          n964 = case shown="假" w1331 {
            tunnel: [w1334 ""] -> w1330
            tunnel: w1322 -> [w1334 _]
            frame False {
              n965 = global read "全局 小时数据发送次数.vi" "小时数据发送次数"() -> (w1333:i32)
              n966 = Increment(x=w1333) -> (x+1=w1332:i32)
              n967 = global write "全局 小时数据发送次数.vi" "小时数据发送次数"(w1332) -> ()
            }
            frame True {
              n968 = global read "全局 小时数据发送次数.vi" "小时数据发送次数"() -> (w1336:i32)
              n969 = Increment(x=w1336) -> (x+1=w1335:i32)
              n970 = global write "全局 小时数据发送次数.vi" "小时数据发送次数"(w1335) -> ()
            }
          }
        }
        frame "返回执行结果" {
        }
      }
    }
    frame "提取仪器参数" {
      n971 = global read "全局1.vi" "枚举"() -> (w1340:enum16{"返回请求应答", "上传数据", "返回执行结果"})
      n972 = case shown="\"上传数据\"" w1340 {
        tunnel: ["QnRtn=1" w1350 "ExeRtn=1"] -> w1341
        tunnel: w1339 -> [_ w1348 _]
        frame "返回请求应答", Default {
          n973 = global read "全局 数据数组大小.vi" "数据数组大小"() -> (w1344:i32)
          n974 = Equal To 0?(x=w1344) -> (x = 0?=w1343:bool)
          n975 = case shown="假" w1343 {
            frame False {
            }
            frame True {
              n976 = global read "全局 小时数据发送次数.vi" "小时数据发送次数"() -> (w1346:i32)
              n977 = Increment(x=w1346) -> (x+1=w1345:i32)
              n978 = global write "全局 小时数据发送次数.vi" "小时数据发送次数"(w1345) -> ()
            }
          }
        }
        frame "上传数据" {
          n979 = call "数据发送组合-20200825 (子VI).vi"("枚举"=T6."提取仪器参数", "插值后的数组元素"=w1348) -> ("字符串"=w1347:string)  [unwired: 9 in]
          n980 = Empty String/Path?(string/path=w1347) -> (empty?=w1351:bool)
          n981 = case shown="假" w1351 {
            tunnel: [w1354 ""] -> w1350
            tunnel: w1347 -> [w1354 _]
            frame False {
              n982 = global read "全局 小时数据发送次数.vi" "小时数据发送次数"() -> (w1353:i32)
              n983 = Increment(x=w1353) -> (x+1=w1352:i32)
              n984 = global write "全局 小时数据发送次数.vi" "小时数据发送次数"(w1352) -> ()
            }
            frame True {
              n985 = global read "全局 小时数据发送次数.vi" "小时数据发送次数"() -> (w1356:i32)
              n986 = Increment(x=w1356) -> (x+1=w1355:i32)
              n987 = global write "全局 小时数据发送次数.vi" "小时数据发送次数"(w1355) -> ()
            }
          }
        }
        frame "返回执行结果" {
        }
      }
    }
    frame "报警信息" {
      n988 = global read "全局 小时数据发送次数.vi" "小时数据发送次数"() -> (w1361:i32)
      n989 = Index Array(array=w1363, index (row)=w1361) -> (element=w1360:string[])  [unwired: 1 in]
      n990 = global read "全局1.vi" "枚举"() -> (w1362:enum16{"返回请求应答", "上传数据", "返回执行结果"})
      n991 = case shown="\"上传数据\"" w1362 {
        tunnel: ["QnRtn=1" w1376 "ExeRtn=1"] -> w1364
        tunnel: w1360 -> [_ _ _]
        tunnel: w1359 -> [_ w1371 _]
        frame "返回请求应答", Default {
          n992 = global read "全局 数据数组大小.vi" "数据数组大小"() -> (w1367:i32)
          n993 = Equal To 0?(x=w1367) -> (x = 0?=w1366:bool)
          n994 = case shown="真" w1366 {
            frame False {
            }
            frame True {
              n995 = global read "全局 小时数据发送次数.vi" "小时数据发送次数"() -> (w1369:i32)
              n996 = Increment(x=w1369) -> (x+1=w1368:i32)
              n997 = global write "全局 小时数据发送次数.vi" "小时数据发送次数"(w1368) -> ()
            }
          }
        }
        frame "上传数据" {
          n998 = call "数据发送组合-20200825 (子VI).vi"("枚举"=T6."报警信息", "插值后的数组元素"=w1371) -> ("字符串"=w1370:string)  [unwired: 9 in]
          n999 = Empty String/Path?(string/path=w1370) -> (empty?=w1377:bool)
          n1000 = String Length(string=w1370) -> (length=w1375:i32)
          n1001 = Decrement(x=w1375) -> (x-1=w1374:i32)
          n1002 = String Subset(string=w1370, length (rest)=w1374) -> (substring=w1373:string)  [unwired: 1 in]
          n1003 = case shown="假" w1377 {
            tunnel: [w1380 ""] -> w1376
            tunnel: w1373 -> [w1380 _]
            frame False {
              n1004 = global read "全局 小时数据发送次数.vi" "小时数据发送次数"() -> (w1379:i32)
              n1005 = Increment(x=w1379) -> (x+1=w1378:i32)
              n1006 = global write "全局 小时数据发送次数.vi" "小时数据发送次数"(w1378) -> ()
            }
            frame True {
              n1007 = global read "全局 小时数据发送次数.vi" "小时数据发送次数"() -> (w1382:i32)
              n1008 = Increment(x=w1382) -> (x+1=w1381:i32)
              n1009 = global write "全局 小时数据发送次数.vi" "小时数据发送次数"(w1381) -> ()
            }
          }
        }
        frame "返回执行结果" {
        }
      }
    }
    frame "系统状态" {
      # ",i12002-Info=0,i12003-Info=100,i12031-Info=0"
      # "DataTime=20100301145000;PolId=w01018,i12001-Info=1,i12003-Info=100"
      # "100  当前模式\n101  CODMn状态  （0待机，1运行）\n102  氨氮状态\n103  总磷状态\n104  总氮状态\n105  CODCr状态\n106  运行周期"
      n1010 = Get Date/Time In Seconds() -> (seconds since 1Jan1904=w1402:timestamp)
      n1011 = Format Date/Time String(time format string (%c)="%Y%m%d%H%M%S" ("时间格式字符串(%c)"), seconds (now)=w1402) -> (date/time string=w1401:string)  [unwired: 1 in]
      n1012 = global read "全局 小时数据发送次数.vi" "小时数据发送次数"() -> (w1389:i32)
      n1013 = global read "全局1.vi" "register values"() -> (w1390:u16[])
      n1014 = Build Array("w00000", "w01019", "w21003", "w21011", "w21001", "w01018") -> (w1392:string[])
      n1015 = Index Array(array=w1392, index=w1389) -> (element=w1391:string)
      n1016 = Index Array(array=w1390, index=w1389) -> (element=w1388:u16)
      n1017 = case shown="1, 默认" w1389 {
        tunnel: w1391 -> [w1407 w1412]
        tunnel: w1388 -> [w1408 _]
        tunnel: [w1405 w1411] -> w1387
        frame 1, Default {
          n1018 = Number To Decimal String(number=w1408) -> (decimal integer string=w1409:string)  [unwired: 1 in]
          n1019 = Format Into String(w1409) -> (resulting string=w1406:string)  [unwired: 3 in, 1 out]
          n1020 = Format Into String(format string="PolId=%s,i12001-Info=%s,i12002-Info=0;" ("格式字符串"), w1407, w1406) -> (resulting string=w1405:string)  [unwired: 2 in, 1 out]
        }
        frame 0 {
          n1021 = Format Into String(format string="PolId=%s,i22001-Info=0,i22002-Info=1,i22003-Info=0;" ("格式字符串"), w1412) -> (resulting string=w1411:string)  [unwired: 2 in, 1 out]
        }
      }
      n1022 = Format Into String(format string="DataTime=%s;%s" ("格式字符串"), w1401, w1387) -> (resulting string=w1398:string)  [unwired: 2 in, 1 out]
      n1023 = String Length(string=w1398) -> (length=w1400:i32)
      n1024 = Decrement(x=w1400) -> (x-1=w1399:i32)
      n1025 = String Subset(string=w1398, length (rest)=w1399) -> (substring=w1397:string)  [unwired: 1 in]
    }
    frame "运行模式" {
      # "DataTime=20100301145000;PolId=w01018,i12001-Info=1,i12003-Info=0"
      # "100  当前模式\n101  CODMn状态  （0待机，1运行）\n102  氨氮状态\n103  总磷状态\n104  总氮状态\n105  CODCr状态\n106  运行周期"
      n1026 = Get Date/Time In Seconds() -> (seconds since 1Jan1904=w1421:timestamp)
      n1027 = Format Date/Time String(time format string (%c)="%Y%m%d%H%M%S" ("时间格式字符串(%c)"), seconds (now)=w1421) -> (date/time string=w1418:string)  [unwired: 1 in]
      n1028 = global read "全局1.vi" "register values"() -> (w1423:u16[])
      n1029 = Index Array(array=w1423, index=0 ("索引")) -> (element=w1415:u16)
      n1030 = Number To Decimal String(number=w1415) -> (decimal integer string=w1417:string)  [unwired: 1 in]
      n1031 = Format Into String(format string="RunMode=%s;" ("格式字符串"), w1417) -> (resulting string=w1414:string)  [unwired: 2 in, 1 out]
      n1032 = Format Into String(format string="DataTime=%s;%s" ("格式字符串"), w1418, w1414) -> (resulting string=w1420:string)  [unwired: 2 in, 1 out]
    }
    frame "测量周期" {
      n1033 = global read "全局1.vi" "register values"() -> (w1434:u16[])
      n1034 = Get Date/Time In Seconds() -> (seconds since 1Jan1904=w1432:timestamp)
      n1035 = Format Date/Time String(time format string (%c)="%Y%m%d%H%M%S" ("时间格式字符串(%c)"), seconds (now)=w1432) -> (date/time string=w1429:string)  [unwired: 1 in]
      n1036 = Index Array(array=w1434, index=6 ("索引")) -> (element=w1426:u16)
      n1037 = Number To Decimal String(number=w1426) -> (decimal integer string=w1427:string)  [unwired: 1 in]
      n1038 = Format Into String(format string="RunInterval=%s;" ("格式字符串"), w1427) -> (resulting string=w1425:string)  [unwired: 2 in, 1 out]
      n1039 = Format Into String(format string="DataTime=%s;%s" ("格式字符串"), w1429, w1425) -> (resulting string=w1431:string)  [unwired: 2 in, 1 out]
    }
    frame "各参数测量周期" {
      # "QN=20101108135153914;ST=21;CN=2084;PW=123456;MN=A110000_0001;Flag=9;CP=&&DataTime=20100301145000;PolId=w01018,RunInterval=4;PolId=w01019,RunInterval=4;...&&"
      n1040 = global read "全局1.vi" "读取各参数测量周期的值"() -> (w1437:u16[])
      n1041 = Get Date/Time In Seconds() -> (seconds since 1Jan1904=w1440:timestamp)
      n1042 = Format Date/Time String(time format string (%c)="%Y%m%d%H%M%S" ("时间格式字符串(%c)"), seconds (now)=w1440) -> (date/time string=w1438:string)  [unwired: 1 in]
      n1043 = call "2084上传各参数测量周期.vi"("读取各参数测量周期的值"=w1437) -> ("字符串"=w1436:string)  [unwired: 10 in]
      n1044 = Format Into String(format string="DataTime=%s;%s" ("格式字符串"), w1438, w1436) -> (resulting string=w1439:string)  [unwired: 2 in, 1 out]
    }
    frame "超标留样" {
      # "DataTime=20100301145000;PolId=w01018,i12001-Info=1,i12003-Info=0"
      # "100  当前模式\n101  CODMn状态  （0待机，1运行）\n102  氨氮状态\n103  总磷状态\n104  总氮状态\n105  CODCr状态\n106  运行周期"
      n1045 = global read "全局1.vi" "register values"() -> (w1452:u16[])
      n1046 = Get Date/Time In Seconds() -> (seconds since 1Jan1904=w1450:timestamp)
      n1047 = Format Date/Time String(time format string (%c)="%Y%m%d%H%M%S" ("时间格式字符串(%c)"), seconds (now)=w1450) -> (date/time string=w1447:string)  [unwired: 1 in]
      n1048 = Index Array(array=w1452, index=7 ("索引")) -> (element=w1444:u16)
      n1049 = Number To Decimal String(number=w1444) -> (decimal integer string=w1445:string)  [unwired: 1 in]
      n1050 = Format Into String(format string="VaseNo=%s;" ("格式字符串"), w1445) -> (resulting string=w1443:string)  [unwired: 2 in, 1 out]
      n1051 = Format Into String(format string="DataTime=%s;%s" ("格式字符串"), w1447, w1443) -> (resulting string=w1449:string)  [unwired: 2 in, 1 out]
    }
  }
  n1052 = case shown="假" w24 {
    tunnel: [w1455 w1459] -> w26
    frame False {
      n1053 = global read "全局1.vi" "枚举"() -> (w1454:enum16{"返回请求应答", "上传数据", "返回执行结果"})
      n1054 = case shown="\"上传数据\"" w1454 {
        tunnel: ["91" ("CN") w1457 "91" ("CN")] -> w1455
        frame "返回请求应答", Default {
        }
        frame "上传数据" {
          n1055 = global read "全局1.vi" "系统编码ST"() -> (w1457:string)
        }
        frame "返回执行结果" {
        }
      }
    }
    frame True {
      n1056 = global read "全局 反控命令枚举.vi" "反控命令枚举"() -> (w1460:enum16{"返回请求应答", "返回执行结果"})
      n1057 = case shown="\"返回执行结果\"" w1460 {
        tunnel: ["91" "91"] -> w1459
        frame "返回请求应答", Default {
        }
        frame "返回执行结果" {
        }
      }
    }
  }
  n1058 = case shown="\"报警信息\", \"采配水仪器参数\", \"操作日志\", \"仪器参数\"" "table输入" {
    tunnel: ["9015" ("ST") w1473 w1481 w1489 w1496 w1503 w1511 w1519 w1528 w1543 w1555 w1563 w1571 w1580 w1589 w1606 w1614 w1622 w1630 w1638 w1646 w1657 w1669 w1681 w1693 w1705 w1713 "3020" ("ST") "3042" ("ST") "3056" ("ST") "2084" ("ST") "3015" ("ST")] -> w29
    tunnel: ["9" ("ST") "9" ("ST") "9" ("ST") "8" ("ST") "8" ("ST") "9" ("ST") "9" ("ST") "9" ("ST") "9" ("ST") "9" ("ST") "11" ("ST") "9" ("ST") "9" ("ST") w1583 "9" ("ST") "9" ("ST") "9" ("ST") "9" ("ST") "9" ("ST") "9" ("ST") "9" ("ST") "9" ("ST") "9" ("ST") "9" ("ST") "9" ("ST") "9" ("ST") "9" ("ST") "9" ("ST") "9" ("ST") "9" ("ST") "9" ("ST") "9" ("ST")] -> w28
    tunnel: w19 -> [_ w1471 w1479 w1490 w1497 w1504 w1512 w1520 w1529 w1545 w1557 w1565 w1573 w1582 w1592 w1608 w1616 w1624 w1632 w1640 w1648 w1659 w1671 w1683 w1695 w1707 w1715 w1721 w1725 w1729 w1733 w1737]
    tunnel: [_ w1471 w1479 w1490 w1497 w1504 w1512 w1520 w1529 w1545 w1557 w1565 w1573 w1582 w1592 w1608 w1616 w1624 w1632 w1640 w1648 w1659 w1671 w1683 w1695 w1707 w1715 w1721 w1725 w1729 w1733 w1737] -> w8
    tunnel: [w1463 w1470 w1478 w1486 w1494 w1501 w1509 w1517 w1525 w1542 w1554 w1562 w1570 w1579 w1591 w1604 w1612 w1620 w1628 w1636 w1644 w1652 w1664 w1676 w1688 w1700 w1712 w1720 w1724 w1728 w1732 w1736] -> w20
    tunnel: [_ _ _ _ _ _ _ _ _ _ w1552 _ _ _ _ _ _ _ _ _ _ _ _ _ _ _ _ _ _ _ _ _] -> w6
    tunnel: [_ _ _ _ _ _ _ _ _ _ w1550 _ _ _ _ _ _ _ _ _ _ _ _ _ _ _ _ _ _ _ _ _] -> w5
    frame "心跳包", Default {
      # "心跳包"
      n1059 = Get Date/Time In Seconds() -> (seconds since 1Jan1904=w1466:timestamp)
      n1060 = Format Date/Time String(time format string (%c)="%Y%m%d%H%M%S%3u" ("时间格式字符串(%c)"), seconds (now)=w1466) -> (date/time string=w1465:string)  [unwired: 1 in]
      n1061 = Search and Replace String(input string=w1465, search string="." ("搜索字符串")) -> (result string=w1463:string)  [unwired: 6 in, 3 out]
    }
    frame "提取数采仪时间" {
      n1062 = global read "全局1.vi" "枚举"() -> (w1474:enum16{"返回请求应答", "上传数据", "返回执行结果"})
      n1063 = case shown="\"返回执行结果\"" w1474 {
        tunnel: ["9011" ("CN") "1014" ("CN") "9012" ("CN")] -> w1473
        frame "返回请求应答", Default {
        }
        frame "上传数据" {
        }
        frame "返回执行结果" {
        }
      }
      n1064 = local read "QN"() -> (w1470:string)
    }
    frame "提取实时数据间隔" {
      n1065 = global read "全局1.vi" "枚举"() -> (w1482:enum16{"返回请求应答", "上传数据", "返回执行结果"})
      n1066 = case shown="\"上传数据\"" w1482 {
        tunnel: ["9011" ("CN") "1061" ("CN") "9012" ("CN")] -> w1481
        frame "返回请求应答", Default {
        }
        frame "上传数据" {
        }
        frame "返回执行结果" {
        }
      }
      n1067 = local read "QN"() -> (w1478:string)
    }
    frame "反控命令" {
      n1068 = global read "全局 反控命令枚举.vi" "反控命令枚举"() -> (w1487:enum16{"返回请求应答", "返回执行结果"})
      n1069 = case shown="\"返回请求应答\", 默认" w1487 {
        tunnel: ["9011" ("CN") "9012" ("CN")] -> w1489
        frame "返回请求应答", Default {
        }
        frame "返回执行结果" {
        }
      }
      n1070 = local read "QN"() -> (w1486:string)
    }
    frame "超标留样返回" {
      n1071 = global read "全局1.vi" "枚举"() -> (w1493:enum16{"返回请求应答", "上传数据", "返回执行结果"})
      n1072 = case shown="\"上传数据\"" w1493 {
        tunnel: ["9011" ("CN") "3015" ("CN") "9012" ("CN")] -> w1496
        frame "返回请求应答", Default {
        }
        frame "上传数据" {
        }
        frame "返回执行结果" {
        }
      }
      n1073 = local read "QN"() -> (w1494:string)
    }
    frame "提取经纬度环境信息" {
      n1074 = global read "全局1.vi" "枚举"() -> (w1505:enum16{"返回请求应答", "上传数据", "返回执行结果"})
      n1075 = case shown="\"上传数据\"" w1505 {
        tunnel: ["9011" ("CN") "3041" ("CN") "9012" ("CN")] -> w1503
        frame "返回请求应答", Default {
        }
        frame "上传数据" {
        }
        frame "返回执行结果" {
        }
      }
      n1076 = local read "QN"() -> (w1501:string)
    }
    frame "提取现场系统信息" {
      n1077 = global read "全局1.vi" "枚举"() -> (w1513:enum16{"返回请求应答", "上传数据", "返回执行结果"})
      n1078 = case shown="\"上传数据\"" w1513 {
        tunnel: ["9011" ("CN") "3040" ("CN") "9012" ("CN")] -> w1511
        frame "返回请求应答", Default {
        }
        frame "上传数据" {
        }
        frame "返回执行结果" {
        }
      }
      n1079 = local read "QN"() -> (w1509:string)
    }
    frame "提取监测仪表时间" {
      n1080 = global read "全局1.vi" "枚举"() -> (w1521:enum16{"返回请求应答", "上传数据", "返回执行结果"})
      n1081 = case shown="\"返回执行结果\"" w1521 {
        tunnel: ["9011" ("CN") "1011" ("CN") "9012" ("CN")] -> w1519
        frame "返回请求应答", Default {
        }
        frame "上传数据" {
        }
        frame "返回执行结果" {
        }
      }
      n1082 = local read "QN"() -> (w1517:string)
    }
    frame "实时数据" {
      n1083 = global read "全局1.vi" "枚举"() -> (w1527:enum16{"返回请求应答", "上传数据", "返回执行结果"})
      n1084 = case shown="\"上传数据\"" w1527 {
        tunnel: ["9011" ("CN") w1532 "9012" ("CN")] -> w1528
        frame "返回请求应答", Default {
        }
        frame "上传数据" {
          n1085 = global read "全局 实时数据参数.vi" "实时数据参数"() -> (w1531:string)
          n1086 = case shown="\"平行样测试\"" w1531 {
            tunnel: ["2011" ("CN") "2064" ("CN") "2082" ("CN") "2063" ("CN") "2062" ("CN") "2065" ("CN") "2066" ("CN") "fff" ("CN")] -> w1532
            frame "水样测试", Default {
            }
            frame "平行样测试" {
            }
            frame "集成干预测试" {
            }
            frame "加标回收测试" {
            }
            frame "核查数据" {
            }
            frame "空白测试" {
            }
            frame "跨度核查" {
            }
            frame "" {
            }
          }
        }
        frame "返回执行结果" {
        }
      }
      n1087 = local read "QN"() -> (w1525:string)
    }
    frame "小时数据" {
      # "监测小时数据"
      n1088 = global read "全局1.vi" "枚举"() -> (w1544:enum16{"返回请求应答", "上传数据", "返回执行结果"})
      n1089 = case shown="\"上传数据\"" w1544 {
        tunnel: ["9011" ("CN") "2061" ("CN") "9012" ("CN")] -> w1543
        frame "返回请求应答", Default {
        }
        frame "上传数据" {
        }
        frame "返回执行结果" {
        }
      }
      n1090 = local read "QN"() -> (w1542:string)
    }
    frame "剖面数据" {
      n1091 = global read "全局1.vi" "枚举"() -> (w1556:enum16{"返回请求应答", "上传数据", "返回执行结果"})
      n1092 = case shown="\"上传数据\"" w1556 {
        tunnel: ["9011" ("CN") "2083" ("CN") "9012" ("CN")] -> w1555
        frame "返回请求应答", Default {
        }
        frame "上传数据" {
        }
        frame "返回执行结果" {
        }
      }
      n1093 = global read "全局 数据数组大小.vi" "当前包号"() -> (w1551:i32)
      n1094 = global read "全局 数据数组大小.vi" "总包数"() -> (w1553:i32)
      n1095 = Number To Decimal String(number=w1553) -> (decimal integer string=w1552:string)  [unwired: 1 in]
      n1096 = Number To Decimal String(number=w1551) -> (decimal integer string=w1550:string)  [unwired: 1 in]
      n1097 = local read "QN"() -> (w1554:string)
    }
    frame "剖面多参数H" {
      # "监测小时数据"
      n1098 = global read "全局1.vi" "枚举"() -> (w1564:enum16{"返回请求应答", "上传数据", "返回执行结果"})
      n1099 = case shown="\"上传数据\"" w1564 {
        tunnel: ["9011" ("CN") "2061" ("CN") "9012" ("CN")] -> w1563
        frame "返回请求应答", Default {
        }
        frame "上传数据" {
        }
        frame "返回执行结果" {
        }
      }
      n1100 = local read "QN"() -> (w1562:string)
    }
    frame "剖面多参数S" {
      # "监测小时数据"
      n1101 = global read "全局1.vi" "枚举"() -> (w1572:enum16{"返回请求应答", "上传数据", "返回执行结果"})
      n1102 = case shown="\"上传数据\"" w1572 {
        tunnel: ["9011" ("CN") "2011" ("CN") "9012" ("CN")] -> w1571
        frame "返回请求应答", Default {
        }
        frame "上传数据" {
        }
        frame "返回执行结果" {
        }
      }
      n1103 = local read "QN"() -> (w1570:string)
    }
    frame "提取小时数据" {
      # "监测小时数据"
      n1104 = global read "全局1.vi" "枚举"() -> (w1581:enum16{"返回请求应答", "上传数据", "返回执行结果"})
      n1105 = global read "断电保存全局.vi" "数据组合发送"() -> (w1578:bool)
      n1106 = case shown="\"上传数据\"" w1581 {
        tunnel: ["9011" ("CN") "2061" ("CN") "9012" ("CN")] -> w1580
        frame "返回请求应答", Default {
        }
        frame "上传数据" {
        }
        frame "返回执行结果" {
        }
      }
      n1107 = case shown="假" w1578 {
        tunnel: ["9" ("ST") "9" ("ST")] -> w1583
        frame False {
        }
        frame True {
        }
      }
      n1108 = local read "QN"() -> (w1579:string)
    }
    frame "提取实时数据" {
      # "提取实时数据"
      n1109 = global read "全局1.vi" "枚举"() -> (w1590:enum16{"返回请求应答", "上传数据", "返回执行结果"})
      n1110 = case shown="\"上传数据\"" w1590 {
        tunnel: ["9011" ("CN") w1596 "9012" ("CN")] -> w1589
        frame "返回请求应答", Default {
        }
        frame "上传数据" {
          n1111 = global read "全局 实时数据参数.vi" "实时数据参数"() -> (w1595:string)
          n1112 = case shown="\"平行样测试\"" w1595 {
            tunnel: ["2011" ("CN") "2064" ("CN") "2063" ("CN") "2065" ("CN") "2066" ("CN") "fff" ("CN")] -> w1596
            frame "水样测试", Default {
            }
            frame "平行样测试" {
            }
            frame "加标回收测试" {
            }
            frame "空白测试" {
            }
            frame "跨度核查" {
            }
            frame "" {
            }
          }
        }
        frame "返回执行结果" {
        }
      }
      n1113 = local read "QN"() -> (w1591:string)
    }
    frame "跨度核查" {
      # "跨度核查"
      n1114 = global read "全局1.vi" "枚举"() -> (w1607:enum16{"返回请求应答", "上传数据", "返回执行结果"})
      n1115 = case shown="\"上传数据\"" w1607 {
        tunnel: ["9011" ("CN") "2066" ("ST") "9012" ("CN")] -> w1606
        frame "返回请求应答", Default {
        }
        frame "上传数据" {
        }
        frame "返回执行结果" {
        }
      }
      n1116 = local read "QN"() -> (w1604:string)
    }
    frame "提取加标回收" {
      # "提取加标回收"
      n1117 = global read "全局1.vi" "枚举"() -> (w1615:enum16{"返回请求应答", "上传数据", "返回执行结果"})
      n1118 = case shown="\"上传数据\"" w1615 {
        tunnel: ["9011" ("CN") "2063" ("ST") "9012" ("CN")] -> w1614
        frame "返回请求应答", Default {
        }
        frame "上传数据" {
        }
        frame "返回执行结果" {
        }
      }
      n1119 = local read "QN"() -> (w1612:string)
    }
    frame "提取平行样" {
      # "提取平行样"
      n1120 = global read "全局1.vi" "枚举"() -> (w1623:enum16{"返回请求应答", "上传数据", "返回执行结果"})
      n1121 = case shown="\"上传数据\"" w1623 {
        tunnel: ["9011" ("CN") "2064" ("ST") "9012" ("CN")] -> w1622
        frame "返回请求应答", Default {
        }
        frame "上传数据" {
        }
        frame "返回执行结果" {
        }
      }
      n1122 = local read "QN"() -> (w1620:string)
    }
    frame "空白测试", "零点核查" {
      # "零点核查"
      n1123 = global read "全局1.vi" "枚举"() -> (w1631:enum16{"返回请求应答", "上传数据", "返回执行结果"})
      n1124 = case shown="\"上传数据\"" w1631 {
        tunnel: ["9011" ("CN") "2065" ("ST") "9012" ("CN")] -> w1630
        frame "返回请求应答", Default {
        }
        frame "上传数据" {
        }
        frame "返回执行结果" {
        }
      }
      n1125 = local read "QN"() -> (w1628:string)
    }
    frame "核查数据" {
      # "核查数据"
      n1126 = global read "全局1.vi" "枚举"() -> (w1639:enum16{"返回请求应答", "上传数据", "返回执行结果"})
      n1127 = case shown="\"上传数据\"" w1639 {
        tunnel: ["9011" ("CN") "2062" ("ST") "9012" ("CN")] -> w1638
        frame "返回请求应答", Default {
        }
        frame "上传数据" {
        }
        frame "返回执行结果" {
        }
      }
      n1128 = local read "QN"() -> (w1636:string)
    }
    frame "提取集成干预" {
      # "核查数据"
      n1129 = global read "全局1.vi" "枚举"() -> (w1647:enum16{"返回请求应答", "上传数据", "返回执行结果"})
      n1130 = case shown="\"上传数据\"" w1647 {
        tunnel: ["9011" ("CN") "2082" ("ST") "9012" ("CN")] -> w1646
        frame "返回请求应答", Default {
        }
        frame "上传数据" {
        }
        frame "返回执行结果" {
        }
      }
      n1131 = local read "QN"() -> (w1644:string)
    }
    frame "报警信息", "采配水仪器参数", "操作日志", "仪器参数" {
      n1132 = global read "全局1.vi" "枚举"() -> (w1658:enum16{"返回请求应答", "上传数据", "返回执行结果"})
      n1133 = case shown="\"上传数据\"" w1658 {
        tunnel: ["9011" ("CN") "3020" ("CN") "9012" ("CN")] -> w1657
        frame "返回请求应答", Default {
        }
        frame "上传数据" {
        }
        frame "返回执行结果" {
        }
      }
      n1134 = Get Date/Time In Seconds() -> (seconds since 1Jan1904=w1655:timestamp)
      n1135 = Format Date/Time String(time format string (%c)="%Y%m%d%H%M%S%3u" ("时间格式字符串(%c)"), seconds (now)=w1655) -> (date/time string=w1654:string)  [unwired: 1 in]
      n1136 = Search and Replace String(input string=w1654, search string="." ("搜索字符串")) -> (result string=w1652:string)  [unwired: 6 in, 3 out]
    }
    frame "3092日志信息" {
      n1137 = global read "全局1.vi" "枚举"() -> (w1670:enum16{"返回请求应答", "上传数据", "返回执行结果"})
      n1138 = case shown="\"上传数据\"" w1670 {
        tunnel: ["9011" ("CN") "3092" ("CN") "9012" ("CN")] -> w1669
        frame "返回请求应答", Default {
        }
        frame "上传数据" {
        }
        frame "返回执行结果" {
        }
      }
      n1139 = Get Date/Time In Seconds() -> (seconds since 1Jan1904=w1667:timestamp)
      n1140 = Format Date/Time String(time format string (%c)="%Y%m%d%H%M%S%3u" ("时间格式字符串(%c)"), seconds (now)=w1667) -> (date/time string=w1666:string)  [unwired: 1 in]
      n1141 = Search and Replace String(input string=w1666, search string="." ("搜索字符串")) -> (result string=w1664:string)  [unwired: 6 in, 3 out]
    }
    frame "3093报警信息" {
      n1142 = global read "全局1.vi" "枚举"() -> (w1682:enum16{"返回请求应答", "上传数据", "返回执行结果"})
      n1143 = case shown="\"上传数据\"" w1682 {
        tunnel: ["9011" ("CN") "3093" ("CN") "9012" ("CN")] -> w1681
        frame "返回请求应答", Default {
        }
        frame "上传数据" {
        }
        frame "返回执行结果" {
        }
      }
      n1144 = Get Date/Time In Seconds() -> (seconds since 1Jan1904=w1679:timestamp)
      n1145 = Format Date/Time String(time format string (%c)="%Y%m%d%H%M%S%3u" ("时间格式字符串(%c)"), seconds (now)=w1679) -> (date/time string=w1678:string)  [unwired: 1 in]
      n1146 = Search and Replace String(input string=w1678, search string="." ("搜索字符串")) -> (result string=w1676:string)  [unwired: 6 in, 3 out]
    }
    frame "3090仪器参数" {
      n1147 = global read "全局1.vi" "枚举"() -> (w1694:enum16{"返回请求应答", "上传数据", "返回执行结果"})
      n1148 = case shown="\"上传数据\"" w1694 {
        tunnel: ["9011" ("CN") "3090" ("CN") "9012" ("CN")] -> w1693
        frame "返回请求应答", Default {
        }
        frame "上传数据" {
        }
        frame "返回执行结果" {
        }
      }
      n1149 = Get Date/Time In Seconds() -> (seconds since 1Jan1904=w1691:timestamp)
      n1150 = Format Date/Time String(time format string (%c)="%Y%m%d%H%M%S%3u" ("时间格式字符串(%c)"), seconds (now)=w1691) -> (date/time string=w1690:string)  [unwired: 1 in]
      n1151 = Search and Replace String(input string=w1690, search string="." ("搜索字符串")) -> (result string=w1688:string)  [unwired: 6 in, 3 out]
    }
    frame "3091校准信息" {
      n1152 = global read "全局1.vi" "枚举"() -> (w1706:enum16{"返回请求应答", "上传数据", "返回执行结果"})
      n1153 = case shown="\"上传数据\"" w1706 {
        tunnel: ["9011" ("CN") "3091" ("CN") "9012" ("CN")] -> w1705
        frame "返回请求应答", Default {
        }
        frame "上传数据" {
        }
        frame "返回执行结果" {
        }
      }
      n1154 = Get Date/Time In Seconds() -> (seconds since 1Jan1904=w1703:timestamp)
      n1155 = Format Date/Time String(time format string (%c)="%Y%m%d%H%M%S%3u" ("时间格式字符串(%c)"), seconds (now)=w1703) -> (date/time string=w1702:string)  [unwired: 1 in]
      n1156 = Search and Replace String(input string=w1702, search string="." ("搜索字符串")) -> (result string=w1700:string)  [unwired: 6 in, 3 out]
    }
    frame "提取仪器参数" {
      n1157 = global read "全局1.vi" "枚举"() -> (w1714:enum16{"返回请求应答", "上传数据", "返回执行结果"})
      n1158 = case shown="\"上传数据\"" w1714 {
        tunnel: ["9011" ("CN") "3020" ("CN") "9012" ("CN")] -> w1713
        frame "返回请求应答", Default {
        }
        frame "上传数据" {
        }
        frame "返回执行结果" {
        }
      }
      n1159 = local read "QN"() -> (w1712:string)
    }
    frame "系统状态" {
      n1160 = local read "QN"() -> (w1720:string)
    }
    frame "运行模式" {
      n1161 = local read "QN"() -> (w1724:string)
    }
    frame "测量周期" {
      n1162 = local read "QN"() -> (w1728:string)
    }
    frame "各参数测量周期" {
      n1163 = local read "QN"() -> (w1732:string)
    }
    frame "超标留样" {
      n1164 = local read "QN"() -> (w1736:string)
    }
  }
  n1165 = Bundle By Name(cluster="数据块", "ST"=w26, "CN"=w29, "FLAG"=w28, "CP"=w8, "QN"=w20, "MN"="MN", "PW"="PW", "PNUM"=w6, "PNO"=w5) -> (w27:T1)
  n1166 = call "HJ212-2017.vi"("PWD？"=FALSE, "数据段"=w27) -> ("通讯包字符串"=w1:string, "通讯包"=→"通讯包":T2)  [unwired: 7 in, 1 out]
  "通讯包字符串" <- w1
  n1167 = String Length(string=w1) -> (length=→"长度":i32)
  "错误常量" <- "错误常量 2"
  "小时数据发送次数" <- 0 ("小时数据发送次数")
  "核查数据发送次数" <- 0 ("核查数据发送次数")
